vi "ETMF_ACP.vi"() -> ()   [LabVIEW 2019]
uses:
  <vilib>/Utility/error.llb/DialogType.ctl
  <vilib>/DAQmx/write.llb/DAQmx Write (Digital Bool 1Line 1Point).vi
  fd73fc79-9649-4217-8a97-07a7e50f329a.vi
  <vilib>/DAQmx/write.llb/DAQmx Write (Counter Frequency 1Chan 1Samp).vi
  df924464-8897-43aa-8929-2e0273e3eba3.vi
  1855413f-7d1b-4c6c-a6c5-1397daead511.vi
  7b2d4e1c-e7fc-4a66-bc21-bd6d40681ed8.vi
  <vilib>/numeric/Random Number (Range) DBL.vi
  <vilib>/DAQmx/miscellaneous.llb/DAQmx Fill In Error Info.vi
  varGlobal.vi
  <vilib>/DAQmx/create/channels.llb/DAQmx Create Channel (CO-Pulse Generation-Frequency).vi
  <vilib>/DAQmx/configure/timing.llb/DAQmx Timing (Implicit).vi
  <vilib>/addons/control/pid/pid.llb/PID (DBL).vi
  <vilib>/addons/control/pid/pid.llb/PID Gain Schedule (DBL).vi
  <vilib>/addons/control/pid/pid.llb/PID Advanced (DBL).vi
  <vilib>/Utility/file.llb/Write Delimited Spreadsheet (string).vi
  <instrlib>/Agilent 34970/Agilent 34970.lvlib
  <resource>/objmgr/daqmx.rc
  <vilib>/addons/control/pid/NI_PID_pid.lvlib
  <instrlib>/Yokogawa WT200 Series/Yokogawa WT200 Series.lvlib
  <instrlib>/Agilent 681x Series/Agilent 681x Series.lvlib
  48f1d8f6-73b3-4136-b681-12122d971459.vi
  <vilib>/ptbypt/NI_PtbyPt.lvlib
panel:
  out "SPs_Filtro":T1
  in  "Res_TempME":bool
  in  "INC_TempME":bool
  in  "ct_TempME":dbl
  in  "vecTempME":dbl[](array[numeric])
  out "ss_ceval":bool
  in  "vec_CEVAL":dbl[](array[numeric])
  in  "Res_CEVAL":bool
  in  "INC_CEVAL":bool
  in  "ct_CEVAL":dbl
  in  "increment":bool
  in  "ct_Estufa":dbl
  in  "vecEstufa":dbl[](array[numeric])
  in  "reset":bool
  out "PV_MI":dbl
  out "SP_Pwr":i32
  out "iter":i32
  out "Msg Erro":string
  out "error out Pt100":errorcluster
  out "error out TC":errorcluster
  in  "Tab Control":T2(tab)
  out "LIM SS":bool
  out "STEADY?":bool
  in  "TBR (min)":u32=10
  in  "Ts":dbl=1.0
  out "Time":dbl=300.0 format="%<%H:%M:%S>t"
  in  "Logfile_Estufa":string="medsForno"
  in  "Estufa_ON":bool=TRUE
  in  "Frequency":dbl=1.0 min=1.0 max=1.0 format="%.6f"
  in  "PID gains":T3={"proportional gain (Kc)"=39.6, "integral time (Ti, min)"=14.617, "derivative time (Td, min)"=0.0} {"derivative time (Td, min)" format="%.3f"; "integral time (Ti, min)" format="%.3f"; "proportional gain (Kc)" format="%.6f"}
  out "Process variable and Setpoint":cluster{"initial PV":dbl, "SP:":dbl}(graph)
  out "MV":dbl(graph)
  in  "SP:":dbl(slide)=60.0 min=0.0 max=0.0 scale=25.0..80.0
  out "PT100_CH9":dbl
  out "PT100_CH4":dbl
  out "Iteration":i32
  out "Duty Cycle":sgl=0.1 min=0.1 max=99.9 format="%#_6f"
  out "PV":dbl
  in  "STOP":bool
  out "Continue":bool
  in  "Manual":bool
  out "Pinv":u16
  out "DCBus":u16
  out "Vel Real":u16
  out "Chart_velo":cluster{"V(A)":dbl, "V(B)":dbl}(graph)
  in  "Tab Control 3":enum32{"Tensões", "Correntes", "Potências"}(tab)
  out "Chart_tensao":T4(graph)
  out "Chart_cur":T5(graph)
  out "Chart_power":T6(graph)
  out "pwr_cluster":T7
  out "cur_cluster":T8
  out "volt_cluster":T9
  in  "Tempo de integração (s)":u32=5 min=1 max=60 step=1
  in  "Realiza medição WT230":bool=TRUE
  in  "Medição contínua? WT230":bool=TRUE
  in  "Parâmetros serial":T10={"Serial VCC"="COM7", "timeout"=2, "baud rate"=600, "flow control"=0, "data bits"=8, "parity"=enum."None", "stop bits"=10, "termination char"=FALSE} {"stop bits" items=["1.0"=10, "1.5"=15, "2.0"=20]; "flow control" items=["None", "XON/XOFF", "RTS/CTS", "XON/XOFF & RTS/CTS", "DTR/DSR", "XON/XOFF & DTR/DSR"]}
  in  "Velocidade (RPM)":u16 min=1000 max=5000 step=100
  in  "Mensagem":T11(ring)=enum."Read power"
  in  "Limite de corrente":dbl min=0.0 max=0.31 step=0.01 format="%.4f"
  in  "Limite de tensão":dbl=24.0 min=0.0 max=36.0 step=0.5 format="%.4f"
  in  "Seta carga":bool
  in  "Enviar velocidade":bool
  in  "Envia mensagem":bool
  in  "Parar motor":bool
  out "Tradução":string
  out "Resposta":string
  in  "Liga Fonte":bool
  out "Corrente de saída":dbl format="%.4f"
  out "Tensão de saída":dbl format="%.4f"
  out "t":dbl
  in  "Logfile_Watt":string="medsWatt"
  in  "Logfile_Freio":string="medsFreio"
  in  "Tab Control 9":enum32{"COMP_EVAL", "POWER MAP"}(tab)
  out "SP_Vel":i32
  out "CP EV ok":bool
  in  "Skip":bool
  in  "bypass":bool
  in  "teste":bool
  in  "Ts MI":dbl=0.1
  out "MV_MI":dbl=5.583364480052211
  out "Condição Atual":string
  in  "Condicao para teste":T12(ring)
  in  "Logfile_ETMI":string="medsETMI"
  in  "Start EV?":bool
  out "Grafico_MI":cluster{"PV_MI":dbl, "MV_ME":sgl}(graph)
  in  "Ganhos PI do Gain Scheduling":T13(array[cluster])=[{"PID Parameters"={"Kc"=0.00026, "  Ti"=0.027, " Td"=0.0}, "Max PV"=490.0}, {"PID Parameters"={"Kc"=0.00027, "  Ti"=0.037, " Td"=0.0}, "Max PV"=690.0}, {"PID Parameters"={"Kc"=0.00019, "  Ti"=0.024, " Td"=0.0}, "Max PV"=900.0}] {"Max PV" format="%#.2f"; "PID Parameters"."Td" format="%#.3g"; "PID Parameters"."Ti" format="%#.3g"; "PID Parameters"."Kc" format="%#.5f"}
  out "Ganho atual do PI MI":T3={"proportional gain (Kc)"=100.0, "integral time (Ti, min)"=0.0, "derivative time (Td, min)"=0.0} {"derivative time (Td, min)" format="%.3f"; "integral time (Ti, min)" format="%.3f"; "proportional gain (Kc)" format="%.5f"}
  out "Graf_MV_MI":dbl(graph)
  out "MV_MIC":dbl format="%.2f"
  out "MV_C5":dbl format="%.2f"
  out "MV_L1":dbl format="%.2f"
  out "MV_C1":dbl format="%.2f"
  in  "Tab Control 10":enum32{"C1", "L1", "C5", "MIC"}(tab)
  in  "Gains_C1":T3={"proportional gain (Kc)"=232.52, "integral time (Ti, min)"=14.8, "derivative time (Td, min)"=0.0} {"derivative time (Td, min)" format="%.3f"; "integral time (Ti, min)" format="%.3f"; "proportional gain (Kc)" format="%.6f"}
  in  "Gains_L1":T3={"proportional gain (Kc)"=302.56, "integral time (Ti, min)"=7.42, "derivative time (Td, min)"=0.0} {"derivative time (Td, min)" format="%.3f"; "integral time (Ti, min)" format="%.3f"; "proportional gain (Kc)" format="%.6f"}
  in  "Gains_C5":T3={"proportional gain (Kc)"=249.72, "integral time (Ti, min)"=4.7, "derivative time (Td, min)"=0.0} {"derivative time (Td, min)" format="%.3f"; "integral time (Ti, min)" format="%.3f"; "proportional gain (Kc)" format="%.6f"}
  in  "Gains_MIC":T3={"proportional gain (Kc)"=259.498, "integral time (Ti, min)"=6.23, "derivative time (Td, min)"=0.0} {"derivative time (Td, min)" format="%.3f"; "integral time (Ti, min)" format="%.3f"; "proportional gain (Kc)" format="%.6f"}
  in  "TBRMF(min)":u32=10
  out "PV_MIC":dbl
  out "MV_ME":sgl=0.1 min=0.1 max=99.9 format="%#_6f"
  in  "Start PMAP?":bool
  in  "Logfile_ETME":string="medsETME"
  in  "Ts ME":dbl=1.0
  out "PW MP ok":bool
  out "STEADY MF?":bool
  out "Final Ensaio":bool
  out "LIM SS MF":bool
  in  "Tab Control 8":enum32{"C1", "L1", "C5", "MIC"}(tab)
  out "GME_C1":cluster{"SP_C1":dbl, "TP 1":dbl, "SP_F":dbl}(graph)
  out "Graf_MV_C1":dbl(graph)
  out "GME_L1":cluster{"SP_L1":dbl, "TP 10":dbl, "SP_F":dbl}(graph)
  out "Graf_MV_L1":dbl(graph)
  out "GME_C5":cluster{"SP_C5":dbl, "TP 12":dbl, "SP_F":dbl}(graph)
  out "Graf_MV_C5":dbl(graph)
  out "GME_MIC":cluster{"SP_MIC":dbl, "TP 13":dbl, "SP_F":dbl}(graph)
  out "Graf_MV_MIC":dbl(graph)
  in  "Tab Control 11":enum32{"C1", "L1", "C5", "MIC"}(tab)
  in  "zF_C1":dbl=0.75 min=0.0 max=1.0 step=0.1
  out "zF_C1_i":dbl(knob)=0.75 min=0.0 max=0.99 step=0.1 scale=0.0..1.0
  in  "SP_C1":dbl=70.0 caption="SP C011:" min=0.0 max=0.0
  in  "zF_L1":dbl=0.75 min=0.0 max=1.0 step=0.1
  out "zF_L1_i":dbl(knob)=0.75 min=0.0 max=0.99 step=0.1 scale=0.0..1.0
  in  "SP_L1":dbl=70.0 caption="SP L100:" min=0.0 max=0.0
  in  "zF_C5":dbl=0.75 min=0.0 max=1.0 step=0.1
  out "zF_C5_i":dbl(knob)=0.75 min=0.0 max=0.99 step=0.1 scale=0.0..1.0
  in  "SP_C5":dbl=70.0 caption="SP C504:" min=0.0 max=0.0
  in  "zF_MIC":dbl=0.75 min=0.0 max=1.0 step=0.1
  out "zF_MIC_i":dbl(knob)=0.75 min=0.0 max=0.99 step=0.1 scale=0.0..1.0
  in  "SP_MIC":dbl=70.0 caption="SP MIC:" min=0.0 max=0.0
  in  "Tab Control 2":enum32{"1-7", "8-15"}(tab)
  out "G. TP 1":cluster{dbl, "index":i32}(graph)
  out "TP 1":dbl
  out "TP 2":dbl
  out "G. TP 2":cluster{dbl, "index":i32}(graph)
  out "G. TP 3":cluster{dbl, "index":i32}(graph)
  out "TP 3":dbl
  out "G. TP 5":cluster{dbl, "index":i32}(graph)
  out "TP 5":dbl
  out "G. TP 6":cluster{dbl, "index":i32}(graph)
  out "TP 6":dbl
  out "G. TP 7":cluster{dbl, "index":i32}(graph)
  out "TP 7":dbl
  out "G. TP 8":cluster{dbl, "index":i32}(graph)
  out "TP 8":dbl
  out "G. TP 10":cluster{dbl, "index":i32}(graph)
  out "TP 10":dbl
  out "G. TP 11":cluster{dbl, "index":i32}(graph)
  out "TP 11":dbl
  out "G. TP 12":cluster{dbl, "index":i32}(graph)
  out "TP 12":dbl
  out "G. TP 13":cluster{dbl, "index":i32}(graph)
  out "TP 13":dbl
  out "G. TP 15":cluster{dbl, "index":i32}(graph)
  out "TP 15":dbl
  in  "Logfile_TPs":string="medsETMA"
  in  "Logfile_Dina":string="medsYDin"
  out "Chart Temperatura":cluster{dbl, dbl, dbl, dbl, dbl, dbl}(graph)={21.505, 22.941, 24.092, 23.94, 23.972, 20.648}
  out "temp pts":T14
  in  "Tab Control 5":enum32{"CONFIG", "COM"}(tab)
  in  "Configurações":T15={"Tipo de tensão"=enum."AC", "Tensão (V)"=0.0, "Limite de corrente (A)"=0.0, "Frequência (Hz)"=60.0, "Limite de Potência (kW)"=0.0} {"Limite de Potência (kW)" min=0.0 max=300.0; "Frequência (Hz)" min=43.0 max=63.0; "Limite de corrente (A)" min=0.0 max=15.5; "Tensão (V)" min=0.0 max=300.0}
  in  "VISA name (EEC)":refnum<visa-resource-name>="Extech"
  in  "Timeout":i32=10000
  in  "RST*":bool
  in  "error in (EEC)":errorcluster
  out "error Out (EEC)":errorcluster
  in  "Logfile_EEC":string="medsZeec"
  in  "Tab Control 7":enum32{"VOLT", "CURR", "PWR"}(tab)
  out "EEC_VOLT":cluster{"Peak Current":dbl}(graph)
  out "EEC_CURR":cluster{"Peak Current":dbl}(graph)
  out "EEC_PWR":cluster{"Peak Current":dbl}(graph)
  in  "Tab Control 6":enum32{"VOLT", "CURR", "PWR"}(tab)
  out "ACP_VOLT":cluster{"Peak Current":dbl}(graph)
  out "ACP_CUR":T16(graph)
  out "ACP_PWR":T17(graph)
  out "PwrMeas":cluster{"Total Power":dbl, "Power Factor":dbl}
  out "VolMeas":cluster{"AC + DC RMS Voltage":dbl}
  out "CurMeas":T18
  in  "Tab Control 4":enum32{"CONFIG", "PROT", "COM"}(tab)
  in  "Muda tensao":bool
  in  "Triggered Voltage Amplitude (V)":dbl=1.0 min=0.0 max=300.0 format="%#.4g"
  in  "Trigger Delay (s)":dbl=10.0 format="%#.5g"
  in  "Period (s)":dbl=10.0 format="%#.4g"
  in  "Pulse Characteristic":u16(ring) items=["Duty Cycle", "Pulse Width"]
  in  "Pulse Count":dbl=1.0 format="%#.4g"
  in  "Pulse Characteristic Value (%)":dbl=100.0 min=0.0 max=100.0 format="%#.4g"
  in  "Voltage Mode (0: Fix)":u16(ring) items=["Fixed", "Step", "Pulse", "List"]
  in  "Voltage Amplitude (1.0 V)":dbl min=0.0 max=300.0 format="%#.4g"
  in  "RMS Current Limit (1 A)":dbl=0.3 min=0.1 max=10.0 format="%#.4g"
  in  "Peak Current Limit (13 A)":dbl=0.5 min=0.1 max=20.0 format="%#.4g"
  in  "Output Waveform Type (0: Sinusoid)":u16(ring) items=["Sinusoid", "Square", "Clipped Sinusoid", "User Specified"]
  in  "Output Frequency (60 Hz)":dbl=60.0 format="%#.4g"
  in  "Serial Configuration":T19={"Baud Rate"=9600, "Parity"=0, "Data Bits"=8} {"Data Bits" items=["7"=7, "8"=8]; "Parity" items=["None", "Odd", "Even", "Mark", "Space"]; "Baud Rate" items=["300"=300, "600"=600, "1200"=1200, "2400"=2400, "4800"=4800, "9600"=9600]}
  out "error out (6812B)":errorcluster
  in  "VISA  name (6812B)":refnum<visa-resource-name>="6812B"
  in  "Logfile_6812B":string="meds6812B"
  out "EEC_OUT":T20
  # "Controle de Temperatura da Estufa"
  # "Geral"
  # "Respostas do Sistema em Malha Fechada"
  # "Controles"
  # "Medidas"
  # "Freio"
  # "Wattímetro WT230 Yokogawa"
  # "Controles:"
  # "Log File:"
  # "Controles"
  # "Medidas"
  # "Respostas temporais"
  # "Medidas"
  # "Inversor de Frequência"
  # "Controles"
  # "Comandos"
  # "Velocidade atual medida pelo inversor (RPM)"
  # "Tensão de barramento medida pelo inversor (V)"
  # "Parâmetros Serial"
  # "Controle Automático do Ensaio do Térmico"
  # "Log File:"
  # "Condição de Operação"
  # "Medidas do Sistema"
  # "Parâmetros de Controle"
  # "Log File:"
  # "Limites térmicos:"
  # "Amostragem:"
  # "Assentamento:"
  # "Parâmetros de Controle"
  # "Medidas"
  # "Filtro"
  # "+Agressivo"
  # "+Agressivo"
  # "+Agressivo"
  # "+Agressivo"
  # "Temperaturas dos Termopares"
  # "Log file:"
  # "Legenda:"
  # "TP 1: Termopar do Capacitor C011"
  # "TP 3: Termopar do Choke L001"
  # "TP 2: Termopar do Capacitor C009"
  # "TP 5: Termopar do Capacitor C006"
  # "TP 6: Termopar do Fusível F002"
  # "TP 7: Termopar do Conector CN204"
  # "TP 8: Termopar do CI SMPS IC 100"
  # "TP 10: Termopar do Indutor L100"
  # "TP 11: Termopar do Capacitor C112"
  # "TP 12: Termopar do Capacitor C504"
  # "TP 13: Termopar do Microcontrolador IC601"
  # "TP 15: Termopar do Dissipador"
  # "Temperaturas do Motor/Freio"
  # "Log file:"
  # "Fontes de Corrente Alternada Programáveis"
  # "Keysight 6812B"
  # "Medidas:"
  # "Extech EEC-6510"
  # "Medidas:"
  # "Trigger:"
  # "Forma de Onda"
  # "Proteção contra Sobrecorrente"
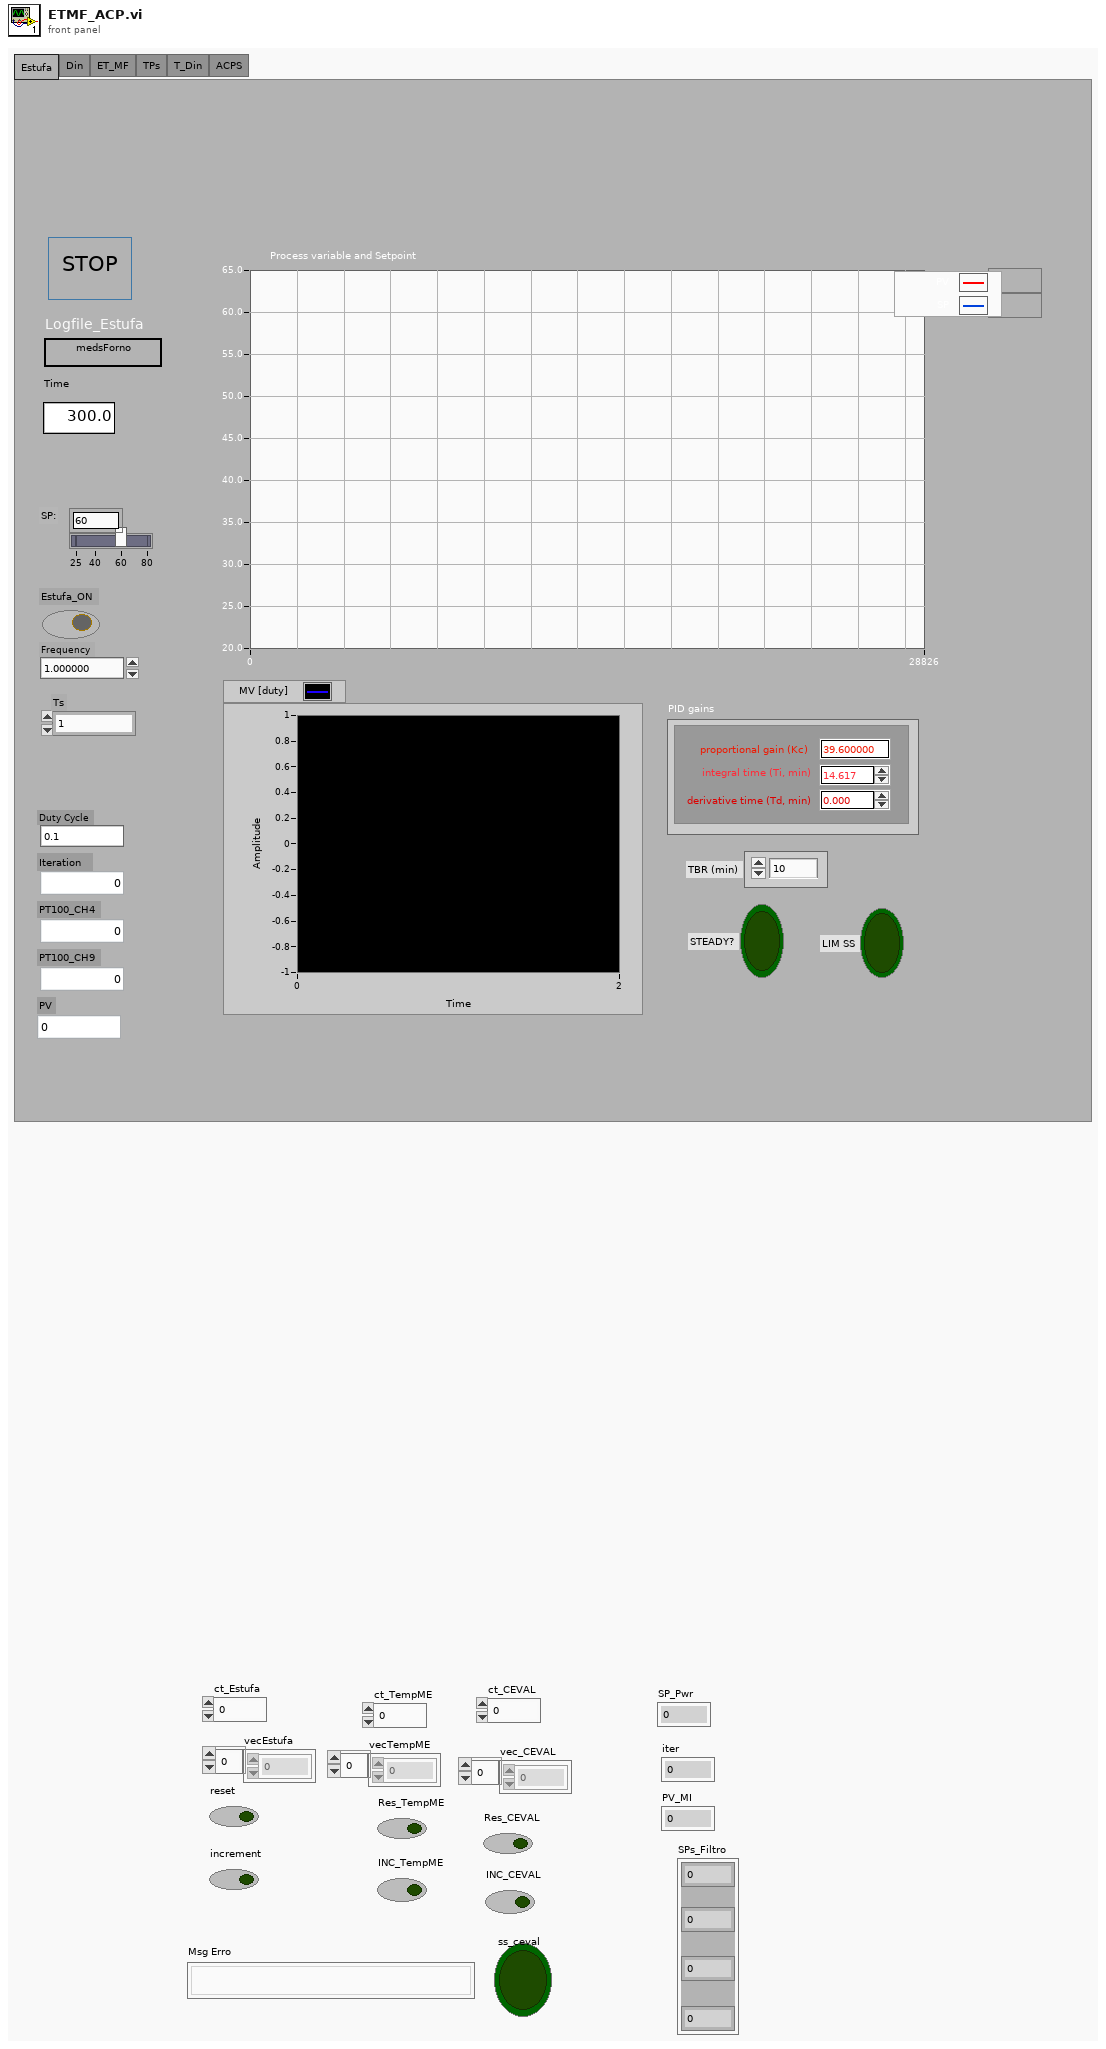
[diagram p1: front panel]
types:
  T1 = cluster{"SP_F":dbl, "SP_F":dbl, "SP_F":dbl, "SP_F":dbl}
  T2 = enum32{"Estufa", "Din", "ET_MF", "TPs", "T_Din", "ACPS"}
  T3 = cluster{"proportional gain (Kc)":dbl, "integral time (Ti, min)":dbl, "derivative time (Td, min)":dbl}
  T4 = cluster{"V(A)":dbl, "V(B)":dbl, "V(E)":dbl, "V(E) 2":dbl}
  T5 = cluster{"I(A)":dbl, "I(B)":dbl, "I(E)":dbl, "I(E) 2":dbl}
  T6 = cluster{"PC(A)":dbl, "PC(B)":dbl, "PC(T)":dbl, "PL(A)":dbl, "PL(B)":dbl, "PL(T)":dbl, "PC(E)":dbl, "PL(E)":dbl, "PL(E) 2":dbl}
  T7 = cluster{"PC(A)":dbl, "PC(B)":dbl, "PC(T)":dbl, "PL(A)":dbl, "PL(B)":dbl, "PL(T)":dbl, "PC(E)":dbl, "PL(E) - 6812B":dbl, "PL(E) - Extech":dbl}
  T8 = cluster{"I(A)":dbl, "I(B)":dbl, "I(E) - 6812B":dbl, "I(E) - Extech":dbl}
  T9 = cluster{"V(A)":dbl, "V(B)":dbl, "V(E) - 6812B":dbl, "V(E) - Extech":dbl}
  T10 = cluster{"Serial VCC":refnum<visa-resource-name>, "timeout":u32, "baud rate":u32, "flow control":u16, "data bits":u16, "parity":enum16{"None", "Odd", "Even", "Mark", "Space"}, "stop bits":u16, "termination char":bool}
  T11 = enum16{"Read set speed", "Read operation status", "Read power", "Read starting trials", "Read bus voltage", "Read temperature", "Read power limitation", "Read PWM mode", "Read PWM frequency", "Read real speed"}
  T12 = enum16{"3500RPM@675W", "3500RPM@720W", "3500RPM@775W", "3500RPM@830W", "3500RPM@885W"}
  T13 = cluster{"PID Parameters":cluster{"Kc":dbl, "  Ti":dbl, " Td":dbl}, "Max PV":dbl}[]
  T14 = cluster{"t1 freio":dbl, "t2 bob 1":dbl, "t5 bob 2":dbl, "t4 estat 2":dbl, "t3 estat 1":dbl, "t6 amb":dbl}
  T15 = cluster{"Tipo de tensão":enum16{"AC", "DC", "AC/DC"}, "Tensão (V)":dbl, "Limite de corrente (A)":dbl, "Frequência (Hz)":dbl, "Limite de Potência (kW)":dbl}
  T16 = cluster{"Peak Current":dbl, "AC RMS Current":dbl}
  T17 = cluster{"Reactive Power":dbl, "Apparent Power":dbl}
  T18 = cluster{"Peak Current":dbl, "AC + DC RMS Cur":dbl}
  T19 = cluster{"Baud Rate":u32, "Parity":u16, "Data Bits":u16}
  T20 = cluster{"Frequency":dbl, "AC Voltage":dbl, "Current":dbl, "Power":dbl, "Power Factor":dbl}
  T21 = enum16{"Start Comm.", "End Comm.", "Wait", "Send Static Message", "Set Speed"}
  T22 = enum8{"Enabled", "Disabled", "Disabled and Grayed Out"}
  T23 = enum16{"Thermocouple", "Thermistor", "RTD", "4-Wire RTD", "Default (Last)"}
  T24 = cluster{"Peak Current":dbl, "AC + DC RMS Current":dbl}
  T25 = cluster{"Frequency":dbl, "AC Voltage":dbl, "Current":dbl, "Power":dbl, "Power Factor":dbl, "Timer":dbl, "a":dbl, "b":dbl, "c ":dbl, "d":dbl, "e":dbl, "f":dbl, "g":dbl}
  T26 = cluster{"Frequency":dbl, "AC Voltage":dbl, "Current":dbl, dbl, "Power Factor":dbl}
  T27 = cluster{"V(A)":dbl, "I(A)":dbl, "V(B)":dbl, "I(B)":dbl, "PC(A)":dbl, "PC(B)":dbl, "PC(T)":dbl, "PL(T)":dbl, "PL(B)":dbl, "PL(A)":dbl, "V(E)":dbl, "PL(E)":dbl, "PC(E)":dbl, "I(E)":dbl, "t":dbl}
  T28 = cluster{"V(A)":dbl, "V(B)":dbl, "V(E)":dbl, "AC Voltage":dbl}
  T29 = cluster{"I(A)":dbl, "I(B)":dbl, "I(E)":dbl, "Current":dbl}
  T30 = cluster{"output":dbl, "output":dbl, "output":dbl, "PL(A)":dbl, "PL(B)":dbl, "PL(T)":dbl, "output":dbl, "PL(E)":dbl, "Power":dbl}
  T31 = typedef "DialogType.ctl" = u16
  T32 = cluster{"TP 1":dbl, "TP 10":dbl, "TP 12":dbl, "TP 13":dbl}
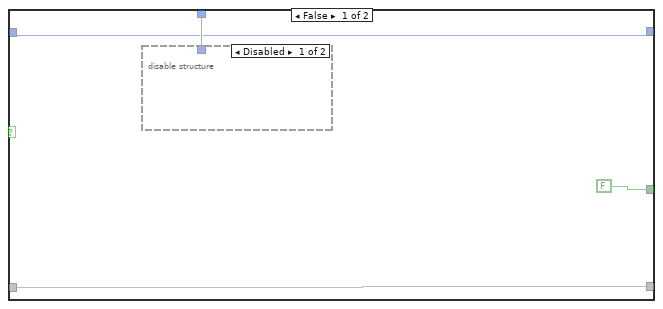
[diagram p2: hidden frame]
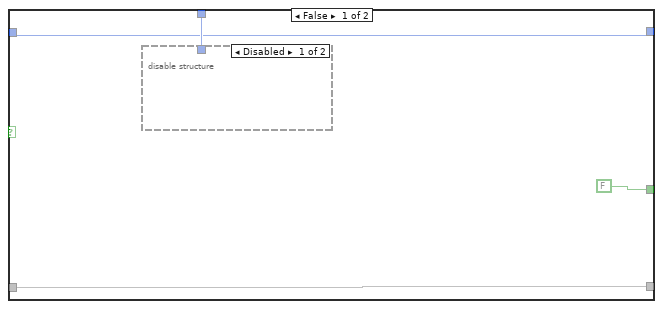
[diagram p4: hidden frame]
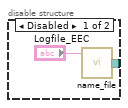
[diagram p9: hidden frame]
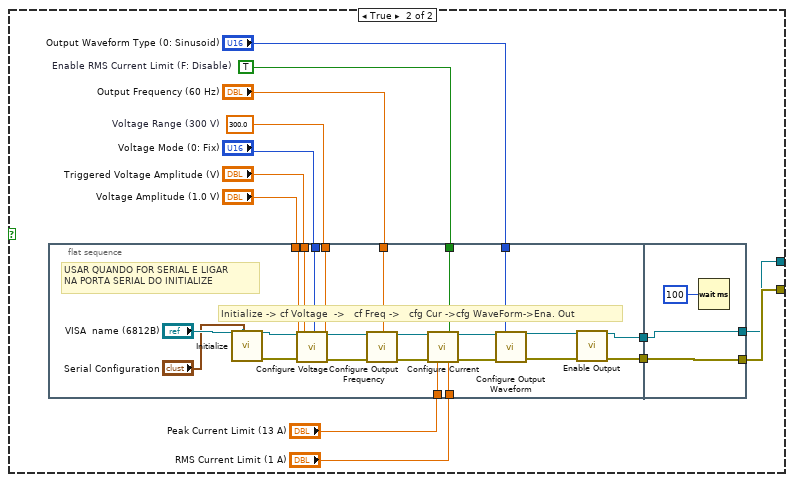
[diagram p11: hidden frame]
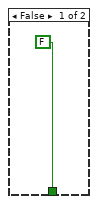
[diagram p12: hidden frame]
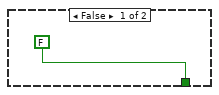
[diagram p13: hidden frame]
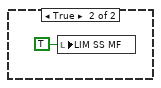
[diagram p17: hidden frame]
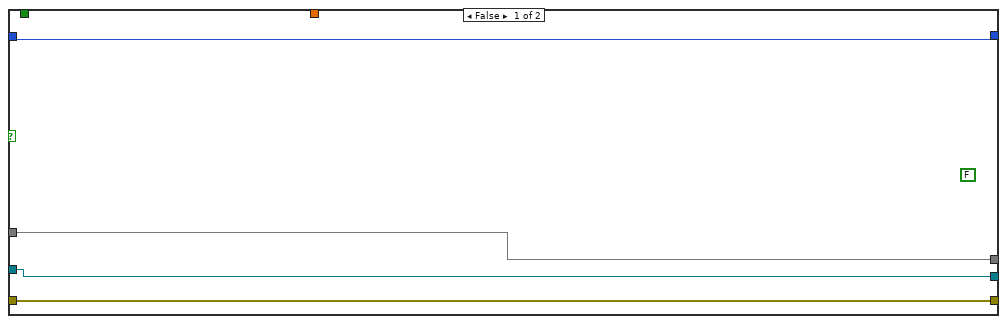
[diagram p18: hidden frame]
diagram:
  # "Se os últimos três valores medidos consecutivamente num intervalo de TBR [minutos] \nestiverem dentro do limite desejado, então a condição é true."
  n1 = flat-sequence {
    tunnel: [w81] -> w14
    tunnel: [w80] -> w13
    tunnel: [w77] -> w12
    tunnel: [w75] -> w11
    tunnel: [w73] -> w10
    tunnel: [w71] -> w9
    tunnel: [w69] -> w8
    tunnel: [w64] -> w7
    tunnel: [w51] -> w6
    tunnel: [w50] -> w5
    tunnel: [w56] -> w4
    tunnel: [w38] -> w3
    tunnel: [w29] -> w2
    tunnel: [w28] -> w1
    tunnel: w14 -> [w302]
    tunnel: w13 -> [w321]
    tunnel: w12 -> [w320]
    tunnel: w11 -> [w315]
    tunnel: w10 -> [w306]
    tunnel: w9 -> [w298]
    tunnel: w8 -> [w296]
    tunnel: w7 -> [w293]
    tunnel: w6 -> [w290]
    tunnel: w5 -> [w289]
    tunnel: w4 -> [w288]
    tunnel: w3 -> [w286]
    tunnel: w2 -> [w271]
    tunnel: w1 -> [w270]
    frame #0 {
      w20 = 0.0 ("Graf_MV_C1")
      w21 = cluster{"SP_C1":dbl, "TP 1":dbl, "SP_F":dbl} {"SP_C1"=0.0, "TP 1"=0.0, "SP_F"=0.0} ("GME_C1")
      w24 = 0.0 ("counter")
      w39 = FALSE ("STOP_GERAL")
      w23 = FALSE ("Auto Enab?")
      w65 = 0.0 ("Temperature 1")
      w22 = 0.0 ("PC(E)")
      w41 = u16 0 ("Velocidade (RPM)")
      w70 = TRUE ("Realiza medição WT230")
      # "Define o tamanho do gauge e do controle do zero do filtro 2 DOF"
      # "Inicia vetor do algoritmo de leituras da estufa e do ceval"
      # "Zera contador do contador de leituras de temp da estufa"
      # "Seta velocidade do motor para o ensaio"
      # "Inicializando as variáveis chart do Wattímetro WT230:"
      # "Inicializando parâmetros controle fonte Lambda:"
      # "Inicializa a fonte Keysight 6812B que liga o ventilador"
      # "Liga fonte Lambda e seta carga para zero"
      # "Estabelece Comunicação com o Inversor"
      # "Inicializando as medidas elétricas da fonte EEC 6510"
      # "Inicializando as medidas elétricas Wattímetro WT330"
      # "Inicializando as variáveis do Agilent 34972A:"
      # "Inicializando as variaveis das malhas de controle da estufa, da carga e das medidores de regime permanente"
      # "Inicializando as medidas elétricas da fonte 6812B"
      # "Inicia Wattímetro e liga relé SSR:"
      # "Controle Automático, Inversor e Fonte  Lambda desligados:"
      # "Zera variaveis lidas pelo inversor e a iteracao"
      # "Declaração variáveis de controle e de erro"
      n2 = case shown="True" TRUE {
        tunnel: [FALSE w228] -> w58
        frame False {
        }
        frame True {
          n3 = flat-sequence {
            tunnel: [w233] -> w229
            tunnel: [w236] -> w230
            tunnel: w229 -> [w236]
            tunnel: [w238] -> w231
            tunnel: w230 -> [w238]
            tunnel: [w241] -> w232
            tunnel: w231 -> [w241]
            tunnel: w232 -> [w246]
            tunnel: [TRUE ("STOP")] -> w228
            frame #0 {
              w234 = refnum<k21> "alimentacao_inversor"  # DAQmx Task Name
              n4 = call <vilib>:"DAQmx Start Task.vi"("task/channels in"=w234) -> ("task out"=w233:refnum<k21>)  [unwired: 13 in, 1 out]
              n5 = call-poly <vilib>:"DAQmx Write.vi"("task/channels in"=w233, "data"=TRUE) -> ()  [unwired: 11 in, 3 out]
            }
            frame #1 {
              # "era 3000"
              n6 = Wait (ms)(milliseconds to wait=u32 100) -> ()  [unwired: 1 out]
            }
            frame #2 {
              # "inicia comunicacao"
              n7 = call "Serial_control.vi"("Função"=T21."Start Comm.", "comm cluster"="Parâmetros serial") -> ()  [unwired: 3 in, 4 out]
            }
            frame #3 {
              # "seta velocidade igual a zero"
              n8 = local read "Parâmetros serial"() -> (w243:T10)
              n9 = call "Serial_control.vi"("Enviar número"=u16 0, "Função"=T21."Set Speed", "comm cluster"=w243) -> ()  [unwired: 2 in, 4 out]
            }
            frame #4 {
              n10 = call <vilib>:"DAQmx Clear Task.vi"("task in"=w246) -> ()  [unwired: 14 in, 1 out]
            }
          }
        }
      }
      n11 = flat-sequence {
        tunnel: [w85] -> w18
        tunnel: [w85] -> w17
        tunnel: [w85] -> w16
        tunnel: [w85] -> w15
        tunnel: w18 -> [w103]
        tunnel: w17 -> [w102]
        tunnel: w16 -> [w100]
        tunnel: w15 -> [w101]
        frame #0 {
          w85 = 1.0
          n12 = disable-structure shown="Disabled" {
            disable-tunnel: [w94 _] -> _
            disable-tunnel: [w91 _] -> _
            disable-tunnel: [w89 _] -> _
            disable-tunnel: [w86 _] -> _
            frame Disabled {
              w88 = 60.0 ("x")
              # "Ti_C1 em seg"
              n13 = local read "Gains_MIC"() -> (w98:T3)
              n14 = local read "Gains_C5"() -> (w97:T3)
              n15 = local read "Gains_C1"() -> (w95:T3)
              n16 = local read "Gains_L1"() -> (w96:T3)
              n17 = Unbundle By Name(w98) -> ("integral time (Ti, min)"=w87:dbl)  [unwired: 1 out]
              n18 = Unbundle By Name(w97) -> ("integral time (Ti, min)"=w90:dbl)  [unwired: 1 out]
              n19 = Unbundle By Name(w95) -> ("integral time (Ti, min)"=w93:dbl)  [unwired: 1 out]
              n20 = Unbundle By Name(w96) -> ("integral time (Ti, min)"=w92:dbl)  [unwired: 1 out]
              n21 = Multiply(x=w88, y=w93) -> (x*y=w94:dbl)
              n22 = Multiply(x=w88, y=w92) -> (x*y=w91:dbl)
              n23 = Multiply(x=w88, y=w90) -> (x*y=w89:dbl)
              n24 = Multiply(x=w88, y=w87) -> (x*y=w86:dbl)
            }
            frame Enabled {
            }
          }
        }
        frame #1 {
          w99 = 0.85 ("zF_C1")
          # "Inicialmente, tau_d = Ti/8"
          # "Control"
          # "Gauge"
          n25 = property on="zF_C1_i" class="Knob (strict)"("Scale.Maximum"=w103) -> ()  [unwired: 2 in, 2 out]
          n26 = property on="zF_L1_i" class="Knob (strict)"("Scale.Maximum"=w102) -> ()  [unwired: 2 in, 2 out]
          n27 = property on="zF_C5_i" class="Knob (strict)"("Scale.Maximum"=w100) -> ()  [unwired: 2 in, 2 out]
          n28 = property on="zF_MIC_i" class="Knob (strict)"("Scale.Maximum"=w101) -> ()  [unwired: 2 in, 2 out]
          n29 = property on="zF_C1" class="DigNum (strict)"("Maximum"=w103) -> ()  [unwired: 2 in, 2 out]
          n30 = property on="zF_L1" class="DigNum (strict)"("Maximum"=w102) -> ()  [unwired: 2 in, 2 out]
          n31 = property on="zF_C5" class="DigNum (strict)"("Maximum"=w100) -> ()  [unwired: 2 in, 2 out]
          n32 = property on="zF_MIC" class="DigNum (strict)"("Maximum"=w101) -> ()  [unwired: 2 in, 2 out]
          n33 = property on="zF_C1" class="DigNum (strict)"("Value"=w99) -> ()  [unwired: 2 in, 2 out]
          n34 = property on="zF_L1" class="DigNum (strict)"("Value"=w99) -> ()  [unwired: 2 in, 2 out]
          n35 = property on="zF_C5" class="DigNum (strict)"("Value"=w99) -> ()  [unwired: 2 in, 2 out]
          n36 = property on="zF_MIC" class="DigNum (strict)"("Value"=w99) -> ()  [unwired: 2 in, 2 out]
        }
      }
      n37 = disable-structure shown="Disabled" {
        disable-tunnel: [w107 _] -> w51
        disable-tunnel: [w106 _] -> w50
        frame Disabled {
          # "Inicializa  e configura a saída da fonte EXTECH 6510 (que alimenta o inversor)"
          n38 = flat-sequence {
            tunnel: [w134] -> w123
            tunnel: [w133] -> w122
            tunnel: [w132] -> w121
            tunnel: [w131] -> w120
            tunnel: [w125] -> w119
            tunnel: w123 -> [w142]
            tunnel: w122 -> [w139]
            tunnel: w121 -> [w141]
            tunnel: w120 -> [w140]
            tunnel: w119 -> [w138]
            tunnel: [w142] -> w118
            tunnel: [w141] -> w117
            tunnel: [w140] -> w116
            tunnel: [w137] -> w115
            tunnel: [w136] -> w114
            tunnel: w118 -> [w147]
            tunnel: w117 -> [w145]
            tunnel: w116 -> [w152]
            tunnel: w115 -> [w153]
            tunnel: w114 -> [w151]
            tunnel: [w144] -> w113
            tunnel: [w143] -> w112
            tunnel: w113 -> [w156]
            tunnel: w112 -> [w155]
            tunnel: [w156] -> w111
            tunnel: [w155] -> w110
            tunnel: w111 -> [w160]
            tunnel: w110 -> [w159]
            tunnel: [w158] -> w109
            tunnel: [w157] -> w108
            tunnel: [w161] -> w106
            tunnel: [w162] -> w107
            tunnel: w109 -> [w162]
            tunnel: w108 -> [w161]
            frame #0 {
              # "Inicializa"
              n39 = Unbundle By Name("Configurações") -> ("Tensão (V)"=w131:dbl, "Limite de corrente (A)"=w132:dbl, "Frequência (Hz)"=w134:dbl)  [unwired: 1 out]
              n40 = call "Inicializa_Reset (SubVI).vi"("error in (no error)"="error in (EEC)", "Reset"="RST*", "Timeout\n(10000 ms)"="Timeout", "VISA Refnum in"="VISA name (EEC)") -> ("error out"=w133:errorcluster, "Mensagem de erro"=→"Msg Erro":string, "VISA Refnum out"=w125:refnum<visa-resource-name>)  [unwired: 4 in, 1 out]
            }
            frame #1 {
              # "Aplica Range de tensão"
              # "Define Range"
              n41 = call "Define_Range (SubVI).vi"("Tensão (V)"=w140) -> ("Range X"=w135:i16)  [unwired: 10 in]
              n42 = call "Range_tensao(SubVI).vi"("error in (no error)"=w139, "Range"=w135, "VISA Refnum in"=w138) -> ("error out"=w137:errorcluster, "VISA Refnum out"=w136:refnum<visa-resource-name>)  [unwired: 7 in]
            }
            frame #2 {
              # "Envia tensão, freq e lim corrente"
              n43 = call "Tensao_AC (SubVI).vi"("error in (no error)"=w153, "Tensão (V)"=w152, "VISA Refnum in"=w151) -> ("error out"=w148:errorcluster, "VISA Refnum out"=w146:refnum<visa-resource-name>)  [unwired: 7 in]
              n44 = call "Frequência (SubVI).vi"("error in (no error)"=w148, "Frequência (Hz)"=w147, "VISA Refnum in"=w146) -> ("error out"=w150:errorcluster, "VISA Refnum out"=w149:refnum<visa-resource-name>)  [unwired: 7 in]
              n45 = call "Limite de corrente High (SubVI).vi"("error in (no error)"=w150, "Limite de corrente"=w145, "VISA Refnum in"=w149) -> ("error out"=w144:errorcluster, "VISA Refnum out"=w143:refnum<visa-resource-name>)  [unwired: 7 in]
            }
            frame #3 {
              n46 = Wait (ms)(milliseconds to wait=u32 500) -> ()  [unwired: 1 out]
            }
            frame #4 {
              # "Liga a saída"
              n47 = call "Power On.vi"("error in (no error)"=w160, "VISA Refnum in"=w159) -> ("error out"=w157:errorcluster, "VISA Refnum out"=w158:refnum<visa-resource-name>)  [unwired: 8 in]
            }
            frame #5 {
            }
          }
        }
        frame Enabled {
        }
      }
      n48 = case shown="True" w58 {
        tunnel: [FALSE ("STOP") w210] -> w52
        frame False {
        }
        frame True {
          n49 = flat-sequence {
            tunnel: [w212] -> w207
            tunnel: [w211] -> w204
            tunnel: [w216] -> w208
            tunnel: w207 -> [w216]
            tunnel: [w215] -> w205
            tunnel: w204 -> [w215]
            tunnel: [w219] -> w209
            tunnel: w208 -> [w219]
            tunnel: [w218] -> w206
            tunnel: w205 -> [w218]
            tunnel: w209 -> [w223]
            tunnel: w206 -> [w222]
            tunnel: [TRUE ("STOP")] -> w210
            frame #0 {
              # "Liga fonte"
              n50 = call <instrlib>:"GENie Config Output On-Off.vi"("Output ON"=TRUE, "VISA"=refnum<visa-resource-name> "Lambda" ("VISA name")) -> ("error out"=w211:errorcluster, "VISA out"=w212:refnum<visa-resource-name>)  [unwired: 8 in]
            }
            frame #1 {
              n51 = Wait (ms)(milliseconds to wait=u32 100) -> ()  [unwired: 1 out]
            }
            frame #2 {
              n52 = local write "Seta carga"(TRUE ("Seta carga")) -> ()
            }
            frame #3 {
              # "corrente igual a zero"
              n53 = call <instrlib>:"GENie Config Current Limit.vi"("error"=w222, "Current Limit"=0.0, "VISA"=w223) -> ()  [unwired: 7 in, 2 out]
            }
            frame #4 {
              n54 = local write "Seta carga"(FALSE ("Seta carga")) -> ()
              n55 = Wait (ms)(milliseconds to wait=u32 100) -> ()  [unwired: 1 out]
            }
            frame #5 {
            }
          }
        }
      }
      n56 = case shown="False" w52 {
        tunnel: [errorcluster {"status"=FALSE, "code"=0, "source"=""} ("error out") w166] -> w29
        tunnel: [w164 w165] -> w28
        frame False {
          n57 = local read "VISA  name (6812B)"() -> (w164:refnum<visa-resource-name>)
        }
        frame True {
          w171 = TRUE  # Enable RMS Current Limit (F: Disable)
          w170 = 300.0  # Voltage Range (300 V)
          n58 = flat-sequence {
            tunnel: "Output Frequency (60 Hz)" -> [w197]
            tunnel: "Voltage Mode (0: Fix)" -> [w195]
            tunnel: "RMS Current Limit (1 A)" -> [w193]
            tunnel: "Output Waveform Type (0: Sinusoid)" -> [w192]
            tunnel: "Voltage Amplitude (1.0 V)" -> [w191]
            tunnel: "Triggered Voltage Amplitude (V)" -> [w190]
            tunnel: w171 -> [w185]
            tunnel: w170 -> [w184]
            tunnel: "Peak Current Limit (13 A)" -> [w181]
            tunnel: [w179] -> w168
            tunnel: [w178] -> w167
            tunnel: w168 -> [w201]
            tunnel: w167 -> [w200]
            tunnel: [w201] -> w165
            tunnel: [w200] -> w166
            frame #0 {
              # "USAR QUANDO FOR SERIAL E LIGAR \nNA PORTA SERIAL DO INITIALIZE"
              # "Initialize -> cf Voltage  ->   cf Freq ->   cfg Cur ->cfg WaveForm->Ena. Out"
              n59 = call <instrlib>:"Initialize.vi"("Serial Configuration"="Serial Configuration", "VISA resource name"="VISA  name (6812B)") -> ("error out"=w196:errorcluster)  [unwired: 8 in, 1 out]
              n60 = call <instrlib>:"Configure Voltage.vi"("VISA resource name"="VISA  name (6812B)", "Triggered Voltage Amplitude (1.0 V)"=w190, "Voltage Range (300 V)"=w184, "Voltage Amplitude (1.0 V)"=w191, "Voltage Mode (0: Fix)"=w195, "error in (no error)"=w196) -> ("VISA resource name out"=w189:refnum<visa-resource-name>, "error out"=w188:errorcluster)  [unwired: 8 in]
              n61 = call <instrlib>:"Configure Output Frequency.vi"("VISA resource name"=w189, "Output Frequency (60 Hz)"=w197, "error in (no error)"=w188) -> ("VISA resource name out"=w198:refnum<visa-resource-name>, "error out"=w199:errorcluster)  [unwired: 11 in]
              n62 = call <instrlib>:"Configure Current.vi"("VISA resource name"=w198, "Enable RMS Current Limit (F: Disable)"=w185, "RMS Current Limit (1 A)"=w193, "error in (no error)"=w199, "Peak Current Limit (13 A)"=w181) -> ("VISA resource name out"=w187:refnum<visa-resource-name>, "error out"=w186:errorcluster)  [unwired: 9 in]
              n63 = call <instrlib>:"Configure Output Waveform.vi"("VISA resource name"=w187, "Output Waveform Type (0: Sinusoid)"=w192, "error in (no error)"=w186) -> ("VISA resource name out"=w183:refnum<visa-resource-name>, "error out"=w182:errorcluster)  [unwired: 11 in]
              n64 = call <instrlib>:"Enable Output.vi"("VISA resource name"=w183, "error in (no error)"=w182) -> ("VISA resource name out"=w179:refnum<visa-resource-name>, "error out"=w178:errorcluster)  [unwired: 12 in]
            }
            frame #1 {
              n65 = Wait (ms)(milliseconds to wait=u32 100) -> ()  [unwired: 1 out]
            }
          }
        }
      }
      n66 = local write "Realiza medição WT230"(w70) -> ()
      n67 = local write "Estufa_ON"(w70) -> ()
      n68 = local write "DCBus"(w41) -> ()
      n69 = local write "Iteration"(w41) -> ()
      n70 = local write "Pinv"(w41) -> ()
      n71 = local write "Velocidade (RPM)"(u16 0 ("Velocidade (RPM)")) -> ()
      n72 = local write "Limite de corrente"(0.0 ("Limite de corrente")) -> ()
      n73 = global write "varGlobal.vi" "STOP_GERAL"(w39) -> ()
      n74 = local write "Enviar velocidade"(w39) -> ()
      n75 = local write "Seta carga"(w39) -> ()
      n76 = local write "Liga Fonte"(w39) -> ()
      n77 = local write "Manual"(w39) -> ()
      n78 = local write "Limite de tensão"(24.0 ("Limite de tensão")) -> ()
      n79 = local write "ct_Estufa"(w24) -> ()
      n80 = Initialize Array(-999.0 ("element"), 3 ("dimension size")) -> (w34:dbl[])
      n81 = local write "vecEstufa"(w34) -> ()
      n82 = local write "ct_CEVAL"(w24) -> ()
      n83 = local write "increment"(w23) -> ()
      n84 = local write "Res_TempME"(w23) -> ()
      n85 = local write "bypass"(w23) -> ()
      n86 = local write "Skip"(w23) -> ()
      n87 = local write "teste"(w23) -> ()
      n88 = local write "reset"(w23) -> ()
      n89 = local write "ct_TempME"(w24) -> ()
      n90 = Initialize Array(-999.0 ("element"), 3 ("dimension size")) -> (w32:dbl[])
      n91 = local write "vec_CEVAL"(w32) -> ()
      n92 = Initialize Array(-999.0 ("element"), 3 ("dimension size")) -> (w27:dbl[])
      n93 = local write "vecTempME"(w27) -> ()
      n94 = disable-structure shown="Disabled" {
        disable-tunnel: [w84 _] -> w69
        frame Disabled {
          n95 = call "name_file.vi"("Identifier"="Logfile_6812B") -> ("appended path"=w84:path)  [unwired: 2 in]
        }
        frame Enabled {
        }
      }
      n96 = disable-structure shown="Enabled" {
        disable-tunnel: [w104 _] -> w56
        frame Disabled {
          n97 = call "name_file.vi"("Identifier"="Logfile_EEC") -> ("appended path"=w104:path)  [unwired: 2 in]
        }
        frame Enabled {
        }
      }
      n98 = call "name_file.vi"("Identifier"="Logfile_ETME") -> ("appended path"=w71:path)  [unwired: 2 in]
      n99 = call <instrlib>:"Initialize.vi"("VISA Resource Name"=refnum<visa-resource-name> "Agilent" ("VISA AGILENT")) -> ("VISA Resource Name Out"=w81:refnum<visa-resource-name>)  [unwired: 13 in, 1 out]
      n100 = call "name_file.vi"("Identifier"="Logfile_Watt") -> ("appended path"=w77:path)  [unwired: 2 in]
      n101 = call "name_file.vi"("Identifier"="Logfile_Estufa") -> ("appended path"=w80:path)  [unwired: 2 in]
      n102 = call "name_file.vi"("Identifier"="Logfile_Freio") -> ("appended path"=w75:path)  [unwired: 2 in]
      n103 = call "name_file.vi"("Identifier"="Logfile_Dina") -> ("appended path"=w64:path)  [unwired: 2 in]
      n104 = call "name_file.vi"("Identifier"="Logfile_TPs") -> ("appended path"=w73:path)  [unwired: 2 in]
      n105 = local write "STOP"(FALSE ("STOP")) -> ()
      n106 = call "name_file.vi"("Identifier"="Logfile_ETMI") -> ("appended path"=w38:path)  [unwired: 2 in]
      "PT100_CH4" <- w65
      "PT100_CH9" <- w65
      "Time" <- w65
      "Duty Cycle" <- sgl 0.01 ("Duty Cycle")
      "PV" <- w22
      "t" <- w22
      "Chart_tensao" <- T4 {"V(A)"=0.0, "V(B)"=0.0, "V(E)"=0.0, "V(E) 2"=0.0} ("Chart_tensao")
      "TP 1" <- w65
      "TP 2" <- w65
      "TP 3" <- w65
      "TP 5" <- w65
      "TP 6" <- w65
      "TP 7" <- w65
      "TP 8" <- w65
      "TP 10" <- w65
      "TP 11" <- w65
      "TP 12" <- w65
      "TP 13" <- w65
      "TP 15" <- w65
      "PV_MIC" <- w22
      "error out (6812B)" <- errorcluster {"status"=FALSE, "code"=0, "source"=""} ("error out")
      "ACP_CUR" <- T16 {"Peak Current"=0.0, "AC RMS Current"=0.0} ("ACP_CUR")
      "ACP_PWR" <- T17 {"Reactive Power"=0.0, "Apparent Power"=0.0} ("ACP_PWR")
      "volt_cluster" <- T4 {"V(A)"=0.0, "V(B)"=0.0, "V(E)"=0.0, "V(E) 2"=0.0} ("volt_cluster")
      "cur_cluster" <- T4 {"V(A)"=0.0, "V(B)"=0.0, "V(E)"=0.0, "V(E) 2"=0.0} ("cur_cluster")
      "pwr_cluster" <- T6 {"PC(A)"=0.0, "PC(B)"=0.0, "PC(T)"=0.0, "PL(A)"=0.0, "PL(B)"=0.0, "PL(T)"=0.0, "PC(E)"=0.0, "PL(E)"=0.0, "PL(E) 2"=0.0} ("pwr_cluster")
      "Chart_power" <- T6 {"PC(A)"=0.0, "PC(B)"=0.0, "PC(T)"=0.0, "PL(A)"=0.0, "PL(B)"=0.0, "PL(T)"=0.0, "PC(E)"=0.0, "PL(E)"=0.0, "PL(E) 2"=0.0} ("Chart_power")
      "Chart_cur" <- T5 {"I(A)"=0.0, "I(B)"=0.0, "I(E)"=0.0, "I(E) 2"=0.0} ("Chart_cur")
      "Chart_velo" <- cluster{"V(A)":dbl, "V(B)":dbl} {"V(A)"=0.0, "V(B)"=0.0} ("Chart_velo")
      "ACP_VOLT" <- cluster{"Peak Current":dbl} {"Peak Current"=0.0} ("ACP_VOLT")
      "EEC_VOLT" <- cluster{"Peak Current":dbl} {"Peak Current"=0.0} ("EEC_VOLT")
      "EEC_CURR" <- cluster{"Peak Current":dbl} {"Peak Current"=0.0} ("EEC_CURR")
      "EEC_PWR" <- cluster{"Peak Current":dbl} {"Peak Current"=0.0} ("EEC_PWR")
      "PW MP ok" <- w23
      "STEADY?" <- w23
      "STEADY MF?" <- w23
      "Final Ensaio" <- w23
      "LIM SS" <- w23
      "LIM SS MF" <- w23
      "Continue" <- w23
      "PV_MI" <- w22
      "CP EV ok" <- w23
      "ss_ceval" <- FALSE ("STEADY_CEVAL")
      "MV_ME" <- w22
      "MV_C1" <- w22
      "MV_L1" <- w22
      "MV_C5" <- w22
      "MV_MIC" <- w22
      "GME_C1" <- w21
      "Graf_MV_C1" <- w20
      "GME_L1" <- w21
      "GME_C5" <- w21
      "GME_MIC" <- w21
      "Graf_MV_L1" <- w20
      "Graf_MV_C5" <- w20
      "Graf_MV_MIC" <- w20
      "SPs_Filtro" <- T1 {"SP_F"=0.0, "SP_F"=0.0, "SP_F"=0.0, "SP_F"=0.0} ("SPs_Filtro")
    }
    frame #1 {
      # "Temporizador"
      n107 = disable-structure shown="Disabled" {
        disable-tunnel: w296 -> [w330 _]
        frame Disabled {
          n108 = call-poly <vilib>:"Write Delimited Spreadsheet.vi"("file path (dialog if empty)"=w330, "1D data"=string[] ["t", "PT[W]", "FP", "IP[A]", "IRMS[A]", "VRMS[V]", "", "", "", "", "", "", ""] ("appended array"), "append to file? (new file:F)"=TRUE, "transpose? (no:F)"=FALSE) -> ("new file path (Not A Path if cancelled)"=w326:path)  [unwired: 10 in, 1 out]
          n109 = while {
            tunnel: w326 -> [w358]
            stop <- w352 stop-if-true
            # "Fator de Potencia"
            # "Tensão AC RMS"
            # "Corrente AC + DC RMS"
            # "Corrente de Pico"
            # "Potência Total"
            # "tempo(s):"
            # "Gerando log das Medidas Elétricas da fonte 6812B"
            n110 = local read "VolMeas"() -> (w347:cluster{"AC + DC RMS Voltage":dbl})
            n111 = local read "PwrMeas"() -> (w344:cluster{"Total Power":dbl, "Power Factor":dbl})
            n112 = local read "CurMeas"() -> (w348:T18)
            n113 = Wait (ms)(milliseconds to wait=u32 25000) -> ()  [unwired: 1 out]
            n114 = Unbundle(w347) -> ("AC + DC RMS Voltage"=w332:dbl)
            n115 = Unbundle(w344) -> ("Total Power"=w338:dbl, "Power Factor"=w337:dbl)
            n116 = Unbundle(w348) -> ("Peak Current"=w335:dbl, "AC + DC RMS Cur"=w334:dbl)
            n117 = Bundle("Total Power"=w338, "Power Factor"=w337) -> (w336:cluster{"Total Power":dbl, "Power Factor":dbl})  [unwired: 1 in]
            n118 = Bundle("AC + DC RMS Voltage"=w332) -> (w331:cluster{"AC + DC RMS Voltage":dbl})  [unwired: 1 in]
            n119 = Bundle("Peak Current"=w335, "AC + DC RMS Cur"=w334) -> (w333:T18)  [unwired: 1 in]
            n120 = local read "t"() -> (w355:dbl)
            n121 = local write "ACP_VOLT"(w331) -> ()
            n122 = local write "ACP_PWR"(w336) -> ()
            n123 = local write "ACP_CUR"(w333) -> ()
            n124 = Number To Exponential String(number=w335, precision (6)=i16 3) -> (E-format string=w341:string)  [unwired: 2 in]
            n125 = Number To Exponential String(number=w334, precision (6)=i16 3) -> (E-format string=w340:string)  [unwired: 2 in]
            n126 = Number To Exponential String(number=w332, precision (6)=i16 3) -> (E-format string=w339:string)  [unwired: 2 in]
            n127 = Number To Exponential String(number=w338, precision (6)=i16 3) -> (E-format string=w345:string)  [unwired: 2 in]
            n128 = Number To Exponential String(number=w337, precision (6)=i16 3) -> (E-format string=w342:string)  [unwired: 2 in]
            n129 = Number To Fractional String(number=w355, precision (6)=i16 3) -> (F-format string=w354:string)  [unwired: 2 in]
            n130 = Build Array(w354, w345, w342, w341, w340, w339) -> (w353:string[])
            n131 = local read "STOP"() -> (w352:bool)
            n132 = call-poly <vilib>:"Write Delimited Spreadsheet.vi"("file path (dialog if empty)"=w358, "1D data"=w353, "append to file? (new file:F)"=TRUE, "transpose? (no:F)"=FALSE) -> ()  [unwired: 10 in, 2 out]
          }
        }
        frame Enabled {
        }
      }
      n133 = while {
        tunnel: w271 -> [w609]
        tunnel: w270 -> [w608]
        stop <- w611 stop-if-true
        n134 = local write "VISA  name (6812B)"(w608) -> ()
        n135 = local write "error out (6812B)"(w609) -> ()
        n136 = local read "STOP"() -> (w611:bool)
        n137 = Wait (ms)(milliseconds to wait=u32 1000) -> ()  [unwired: 1 out]
        n138 = disable-structure shown="Disabled" {
          frame Disabled {
            n139 = call "measPwrCur.vi"() -> ("VolMeas"=w613:cluster{"AC + DC RMS Voltage":dbl}, "CurMeas"=w614:T24, "PwrMeas"=w612:cluster{"Total Power":dbl, "Power Factor":dbl})  [unwired: 4 in, 2 out]
            n140 = local write "PwrMeas"(w612) -> ()
            n141 = local write "CurMeas"(w614) -> ()
            n142 = local write "VolMeas"(w613) -> ()
          }
          frame Enabled {
          }
        }
      }
      n143 = disable-structure shown="Disabled" {
        frame Disabled {
          n144 = call <instrlib>:"Close.vi"() -> ()  [unwired: 11 in, 1 out]
        }
        frame Enabled {
        }
      }
      n145 = disable-structure shown="Disabled" {
        disable-tunnel: w290 -> [w1095 _]
        disable-tunnel: w289 -> [w1094 _]
        frame Disabled {
          n146 = while {
            tunnel: w1095 -> [w1111]
            tunnel: w1094 -> [w1110]
            tunnel: [w1109] -> w1093
            tunnel: [w1099] -> w1092
            stop <- w1108 stop-if-true
            # "kW --> W"
            # "Faz as leituras/medições"
            n147 = local read "Configurações"() -> (w1107:T15)
            n148 = Unbundle By Name(w1107) -> ("Tensão (V)"=w1105:dbl)
            n149 = Wait Until Next ms Multiple(millisecond multiple=u32 1000 ("milliseconds to wait")) -> ()  [unwired: 1 out]
            n150 = call "Is Value Changed.vim"("value"=w1105) -> ("changed or first call?"=w1106:bool)
            n151 = case shown="False" w1106 {
              tunnel: [w1114 w1126] -> w1112
              tunnel: w1111 -> [w1118 w1123]
              tunnel: w1110 -> [w1117 w1122]
              tunnel: [w1115 w1125] -> w1109
              tunnel: [w1116 w1124] -> w1099
              tunnel: w1105 -> [_ w1121]
              frame False {
                n152 = call "Medicao(SubVI).vi"("error in (no error)"=w1117, "VISA Refnum in"=w1118) -> ("error out"=w1115:errorcluster, "All Measurements"=w1114:T25, "VISA Refnum out"=w1116:refnum<visa-resource-name>)  [unwired: 7 in]
              }
              frame True {
                # "8"
                n153 = call "Tensao_AC (SubVI).vi"("error in (no error)"=w1122, "Tensão (V)"=w1121, "VISA Refnum in"=w1123) -> ("error out"=w1119:errorcluster, "VISA Refnum out"=w1120:refnum<visa-resource-name>)  [unwired: 7 in]
                n154 = call "Medicao(SubVI).vi"("error in (no error)"=w1119, "VISA Refnum in"=w1120) -> ("error out"=w1125:errorcluster, "All Measurements"=w1126:T25, "VISA Refnum out"=w1124:refnum<visa-resource-name>)  [unwired: 7 in]
              }
            }
            n155 = Unbundle By Name(w1112) -> ("Frequency"=w1104:dbl, "AC Voltage"=w1103:dbl, "Current"=w1102:dbl, "Power"=w1098:dbl, "Power Factor"=w1101:dbl)
            n156 = Multiply(x=w1098, y=1000.0) -> (x*y=w1096:dbl)
            n157 = Bundle("Frequency"=w1104, "AC Voltage"=w1103, "Current"=w1102, w1096, "Power Factor"=w1101) -> (→"EEC_OUT":T26)  [unwired: 1 in]
            n158 = local read "STOP"() -> (w1108:bool)
          }
          n159 = VISA Close(VISA resource name=w1092, error in (no error)=w1093) -> ()  [unwired: 1 out]
        }
        frame Enabled {
        }
      }
      n160 = disable-structure shown="Disabled" {
        disable-tunnel: w288 -> [w1060 _]
        frame Disabled {
          n161 = call-poly <vilib>:"Write Delimited Spreadsheet.vi"("file path (dialog if empty)"=w1060, "1D data"=string[] ["t", "FREQ[Hz]", "VAC[V]", "IOUT[A]", "VRMS[V]", "POUT[W]", "FP", "", "", "", "", "", ""] ("appended array"), "append to file? (new file:F)"=TRUE, "transpose? (no:F)"=FALSE) -> ("new file path (Not A Path if cancelled)"=w1059:path)  [unwired: 10 in, 1 out]
          n162 = while {
            tunnel: w1059 -> [w1070]
            stop <- w1091 stop-if-true
            # "Fator de Potência"
            # "Potência(W):"
            # "Corrente (A)"
            # "Tensão AC (V):"
            # "Frequencia(Hz):"
            # "tempo(s):"
            n163 = local read "EEC_OUT"() -> (w1090:T20)
            n164 = Unbundle By Name(w1090) -> ("Frequency"=w1081:dbl, "AC Voltage"=w1068:dbl, "Current"=w1067:dbl, "Power"=w1064:dbl, "Power Factor"=w1080:dbl)
            n165 = Wait (ms)(milliseconds to wait=u32 1000) -> ()  [unwired: 1 out]
            n166 = Bundle("Power"=w1064) -> (w1065:cluster{"Power":dbl})  [unwired: 1 in]
            n167 = Bundle("AC Voltage"=w1068) -> (w1069:cluster{"AC Voltage":dbl})  [unwired: 1 in]
            n168 = Bundle("Current"=w1067) -> (w1066:cluster{"Current":dbl})  [unwired: 1 in]
            n169 = local write "EEC_PWR"(w1065) -> ()
            n170 = local write "EEC_CURR"(w1066) -> ()
            n171 = local write "EEC_VOLT"(w1069) -> ()
            n172 = local read "t"() -> (w1087:dbl)
            n173 = Number To Fractional String(number=w1087, precision (6)=i16 3) -> (F-format string=w1079:string)  [unwired: 2 in]
            n174 = Number To Fractional String(number=w1081, precision (6)=i16 3) -> (F-format string=w1078:string)  [unwired: 2 in]
            n175 = Number To Fractional String(number=w1068, precision (6)=i16 3) -> (F-format string=w1077:string)  [unwired: 2 in]
            n176 = Number To Fractional String(number=w1067, precision (6)=i16 3) -> (F-format string=w1076:string)  [unwired: 2 in]
            n177 = Number To Fractional String(number=w1064, precision (6)=i16 3) -> (F-format string=w1075:string)  [unwired: 2 in]
            n178 = Number To Fractional String(number=w1080, precision (6)=i16 3) -> (F-format string=w1074:string)  [unwired: 2 in]
            n179 = local read "STOP"() -> (w1091:bool)
            n180 = Build Array(w1079, w1078, w1077, w1076, w1075, w1074) -> (w1071:string[])
            n181 = call-poly <vilib>:"Write Delimited Spreadsheet.vi"("file path (dialog if empty)"=w1070, "1D data"=w1071, "append to file? (new file:F)"=TRUE, "transpose? (no:F)"=FALSE) -> ()  [unwired: 10 in, 2 out]
          }
        }
        frame Enabled {
        }
      }
      n182 = while {
        shift-right: [w617] -> _
        shift-left: T11."Read power" ("Message") -> [w618]
        stop <- w616 stop-if-true
        # "Loop para adquirir as medidas do inversor (tensao barramento, potencia entrada e velocidade real)"
        n183 = case shown="\"Read power\"" w618 {
          tunnel: [T11."Read bus voltage" ("Message") T11."Read real speed" ("Message") T11."Read operation status" ("Message") T11."Read power" ("Message")] -> w617
          frame "Read power" {
            w622 = 0 ("offset")
            # "Manda msg para ler valor da potencia do inversor"
            n184 = local read "Parâmetros serial"() -> (w624:T10)
            n185 = Wait (ms)(milliseconds to wait=u32 10) -> ()  [unwired: 1 out]
            n186 = call "Serial_control.vi"("Message"=T11."Read power", "Função"=T21."Send Static Message", "comm cluster"=w624) -> ("translated message"=w625:string)  [unwired: 2 in, 3 out]
            n187 = local write "Tradução"(w625) -> ()
            n188 = Decimal String To Number(string=w625, offset=w622, default (0L)=w622) -> (number=w626:i32)  [unwired: 1 out]
            n189 = local write "Pinv"(w626) -> ()
          }
          frame "Read bus voltage" {
            w631 = 0 ("offset")
            # "Manda msg para ler valor do BUS DC"
            n190 = local read "Parâmetros serial"() -> (w632:T10)
            n191 = Wait (ms)(milliseconds to wait=u32 10) -> ()  [unwired: 1 out]
            n192 = call "Serial_control.vi"("Message"=T11."Read bus voltage", "Função"=T21."Send Static Message", "comm cluster"=w632) -> ("translated message"=w633:string)  [unwired: 2 in, 3 out]
            n193 = local write "Tradução"(w633) -> ()
            n194 = Decimal String To Number(string=w633, offset=w631, default (0L)=w631) -> (number=w634:i32)  [unwired: 1 out]
            n195 = local write "DCBus"(w634) -> ()
          }
          frame "Read real speed" {
            w640 = 0 ("offset")
            # "Manda msg para ler valor de velocidade real"
            n196 = local read "Parâmetros serial"() -> (w641:T10)
            n197 = Wait (ms)(milliseconds to wait=u32 10) -> ()  [unwired: 1 out]
            n198 = call "Serial_control.vi"("Message"=T11."Read real speed", "Função"=T21."Send Static Message", "comm cluster"=w641) -> ("translated message"=w635:string)  [unwired: 2 in, 3 out]
            n199 = local write "Tradução"(w635) -> ()
            n200 = Decimal String To Number(string=w635, offset=w640, default (0L)=w640) -> (number=w642:i32)  [unwired: 1 out]
            n201 = local write "Vel Real"(w642) -> ()
          }
          frame "Read set speed", "Read operation status", "Read starting trials", "Read temperature".."Read PWM frequency" {
            n202 = Wait (ms)(milliseconds to wait=u32 1) -> ()  [unwired: 1 out]
          }
        }
        n203 = local read "STOP"() -> (w616:bool)
        n204 = Wait (ms)(milliseconds to wait=u32 1000) -> ()  [unwired: 1 out]
      }
      n205 = call-poly <vilib>:"Write Delimited Spreadsheet.vi"("file path (dialog if empty)"=w298, "1D data"=string[] ["t", "SP_C1 [ºC]", "MV_C1 [W]", "SP_L1 [ºC]", "MV_L1 [W]", "SP_C5 [ºC]", "MV_C5 [W]", "SP_MIC [ºC]", "MV_MIC [W]", "MV_ME [W]", "SPF_C1[°C]", "SPF_L1[°C]", "SPF_C5[°C]", "SPF_MIC[°C]"] ("appended array"), "append to file? (new file:F)"=TRUE, "transpose? (no:F)"=FALSE) -> ("new file path (Not A Path if cancelled)"=w297:path)  [unwired: 10 in, 1 out]
      n206 = call-poly <vilib>:"Write Delimited Spreadsheet.vi"("file path (dialog if empty)"=w321, "1D data"=string[] ["t", "PV [ºC]", "SP [ºC]", "MV[%] "] ("appended array"), "append to file? (new file:F)"=TRUE, "transpose? (no:F)"=FALSE) -> ("new file path (Not A Path if cancelled)"=w322:path)  [unwired: 10 in, 1 out]
      n207 = call-poly <vilib>:"Write Delimited Spreadsheet.vi"("file path (dialog if empty)"=w320, "1D data"=string[] ["t", "PL(A)", "PL(B)", "PL(T)", "PL(E)", "V(A)", "V(B)", "V(E)", "I(A)", "I(B)", "I(E)"] ("appended array"), "append to file? (new file:F)"=TRUE, "transpose? (no:F)"=FALSE) -> ("new file path (Not A Path if cancelled)"=w316:path)  [unwired: 10 in, 1 out]
      n208 = call-poly <vilib>:"Write Delimited Spreadsheet.vi"("file path (dialog if empty)"=w315, "1D data"=string[] ["t", "IF", "IR", "VF", "VR", "VelSP", "VelRE", "DCbus", "PINV"] ("appended array"), "append to file? (new file:F)"=TRUE, "transpose? (no:F)"=FALSE) -> ("new file path (Not A Path if cancelled)"=w311:path)  [unwired: 10 in, 1 out]
      n209 = call-poly <vilib>:"Write Delimited Spreadsheet.vi"("file path (dialog if empty)"=w293, "1D data"=string[] ["t", "T_FR", "T_B1", "T_B2", "T_E2", "T_E1", "T_AMB"] ("appended array"), "append to file? (new file:F)"=TRUE, "transpose? (no:F)"=FALSE) -> ("new file path (Not A Path if cancelled)"=w291:path)  [unwired: 10 in, 1 out]
      n210 = call-poly <vilib>:"Write Delimited Spreadsheet.vi"("file path (dialog if empty)"=w306, "1D data"=string[] ["t", "TP1", "TP2", "TP3", "TP5", "TP6", "TP7", "TP8", "TP10", "TP11", "TP12", "TP13", "TP15"] ("appended array"), "append to file? (new file:F)"=TRUE, "transpose? (no:F)"=FALSE) -> ("new file path (Not A Path if cancelled)"=w305:path)  [unwired: 10 in, 1 out]
      n211 = call-poly <vilib>:"Write Delimited Spreadsheet.vi"("file path (dialog if empty)"=w286, "1D data"=string[] ["t", "PV [W]", "SP [W]", "MV[I]"] ("appended array"), "append to file? (new file:F)"=TRUE, "transpose? (no:F)"=FALSE) -> ("new file path (Not A Path if cancelled)"=w282:path)  [unwired: 10 in, 1 out]
      n212 = call <vilib>:"High Resolution Relative Seconds.vi"() -> ("relative seconds"=w310:dbl)
      n213 = while {
        tunnel: w297 -> [w1276]
        stop <- w1265 stop-if-true
        # "SP filtrado PI-MIC"
        # "SP filtrado PI-C5"
        # "SP filtrado PI-L1"
        # "SP filtrado PI-C1"
        # "MV controlador override"
        # "Referencia do MIC"
        # "MV controlador de MIC"
        # "Referencia Cap C5"
        # "MV controlador de C5"
        # "Referencia ind L1"
        # "MV controlador de L1"
        # "tempo(s):"
        # "Referencia Cap C1"
        # "MV controlador de C1"
        # "Gerando log do Controle do Ensaio Térmico para Malha Externa"
        n214 = local read "Ts ME"() -> (w1230:dbl)
        n215 = local read "SPs_Filtro"() -> (w1239:T1)
        n216 = Multiply(x=w1230, y=u32 1000 ("milliseconds to wait")) -> (x*y=w1228:dbl)
        n217 = local read "MV_L1"() -> (w1264:dbl)
        n218 = local read "MV_MIC"() -> (w1256:dbl)
        n219 = local read "MV_C5"() -> (w1257:dbl)
        n220 = local read "SP_L1"() -> (w1262:dbl)
        n221 = local read "SP_MIC"() -> (w1254:dbl)
        n222 = local read "MV_C1"() -> (w1268:dbl)
        n223 = local read "SP_C5"() -> (w1259:dbl)
        n224 = local read "SP_C1"() -> (w1274:dbl)
        n225 = local read "MV_ME"() -> (w1251:sgl)
        n226 = Unbundle(w1239) -> ("SP_F"=w1238:dbl, "SP_F"=w1237:dbl, "SP_F"=w1236:dbl, "SP_F"=w1235:dbl)
        n227 = local read "t"() -> (w1272:dbl)
        n228 = Wait (ms)(milliseconds to wait=w1228) -> ()  [unwired: 1 out]
        n229 = Number To Fractional String(number=w1262, precision (6)=i16 3) -> (F-format string=w1250:string)  [unwired: 2 in]
        n230 = Number To Fractional String(number=w1264, precision (6)=i16 3) -> (F-format string=w1249:string)  [unwired: 2 in]
        n231 = Number To Fractional String(number=w1259, precision (6)=i16 3) -> (F-format string=w1248:string)  [unwired: 2 in]
        n232 = Number To Fractional String(number=w1257, precision (6)=i16 3) -> (F-format string=w1247:string)  [unwired: 2 in]
        n233 = Number To Fractional String(number=w1272, precision (6)=i16 3) -> (F-format string=w1271:string)  [unwired: 2 in]
        n234 = Number To Fractional String(number=w1274, precision (6)=i16 3) -> (F-format string=w1270:string)  [unwired: 2 in]
        n235 = Number To Fractional String(number=w1268, precision (6)=i16 3) -> (F-format string=w1266:string)  [unwired: 2 in]
        n236 = Number To Fractional String(number=w1254, precision (6)=i16 3) -> (F-format string=w1246:string)  [unwired: 2 in]
        n237 = Number To Fractional String(number=w1256, precision (6)=i16 3) -> (F-format string=w1245:string)  [unwired: 2 in]
        n238 = Number To Fractional String(number=w1251, precision (6)=i16 3) -> (F-format string=w1244:string)  [unwired: 2 in]
        n239 = Number To Fractional String(number=w1238, precision (6)=i16 3) -> (F-format string=w1234:string)  [unwired: 2 in]
        n240 = Number To Fractional String(number=w1237, precision (6)=i16 3) -> (F-format string=w1233:string)  [unwired: 2 in]
        n241 = Number To Fractional String(number=w1236, precision (6)=i16 3) -> (F-format string=w1232:string)  [unwired: 2 in]
        n242 = Number To Fractional String(number=w1235, precision (6)=i16 3) -> (F-format string=w1231:string)  [unwired: 2 in]
        n243 = Build Array(w1271, w1270, w1266, w1250, w1249, w1248, w1247, w1246, w1245, w1244, w1234, w1233, w1232, w1231) -> (w1267:string[])
        n244 = local read "STOP"() -> (w1265:bool)
        n245 = call-poly <vilib>:"Write Delimited Spreadsheet.vi"("file path (dialog if empty)"=w1276, "1D data"=w1267, "append to file? (new file:F)"=TRUE, "transpose? (no:F)"=FALSE) -> ()  [unwired: 10 in, 2 out]
      }
      n246 = while {
        tunnel: w282 -> [w868]
        stop <- w853 stop-if-true
        # "tempo(s):"
        # "Saída (PV):"
        # "Referencia (SP):"
        # "sinal de controle (mv):"
        # "Gerando log do Controle do Ensaio Térmico para Malha Interna"
        n247 = local read "MV_MI"() -> (w864:dbl)
        n248 = local read "SP_Pwr"() -> (w857:i32)
        n249 = local read "PV_MI"() -> (w863:dbl)
        n250 = local read "Time"() -> (w861:dbl)
        n251 = Number To Exponential String(number=w864, precision (6)=i16 6) -> (E-format string=w866:string)  [unwired: 2 in]
        n252 = Number To Fractional String(number=w861, precision (6)=i16 6) -> (F-format string=w860:string)  [unwired: 2 in]
        n253 = Number To Fractional String(number=w863, precision (6)=i16 6) -> (F-format string=w859:string)  [unwired: 2 in]
        n254 = Number To Fractional String(number=w857, precision (6)=i16 6) -> (F-format string=w855:string)  [unwired: 2 in]
        n255 = Build Array(w860, w859, w855, w866) -> (w856:string[])
        n256 = local read "STOP"() -> (w853:bool)
        n257 = call-poly <vilib>:"Write Delimited Spreadsheet.vi"("file path (dialog if empty)"=w868, "1D data"=w856, "append to file? (new file:F)"=TRUE, "transpose? (no:F)"=FALSE) -> ()  [unwired: 10 in, 2 out]
        n258 = Wait Until Next ms Multiple(millisecond multiple=u32 100 ("milliseconds to wait")) -> ()  [unwired: 1 out]
      }
      n259 = while {
        tunnel: w322 -> [w1582]
        stop <- w1567 stop-if-true
        # "tempo(s):"
        # "Saída (PV):"
        # "Referencia (SP):"
        # "sinal de controle (mv):"
        # "Gerando log do Controle de Temperatura da Estufa"
        n260 = local read "Duty Cycle"() -> (w1579:sgl)
        n261 = Wait (ms)(milliseconds to wait=u32 1000) -> ()  [unwired: 1 out]
        n262 = local read "SP:"() -> (w1572:dbl)
        n263 = local read "PV"() -> (w1578:dbl)
        n264 = local read "t"() -> (w1576:dbl)
        n265 = Number To Fractional String(number=w1576, precision (6)=i16 3) -> (F-format string=w1575:string)  [unwired: 2 in]
        n266 = Number To Fractional String(number=w1578, precision (6)=i16 3) -> (F-format string=w1574:string)  [unwired: 2 in]
        n267 = Number To Fractional String(number=w1572, precision (6)=i16 3) -> (F-format string=w1570:string)  [unwired: 2 in]
        n268 = Number To Exponential String(number=w1579, precision (6)=i16 3) -> (E-format string=w1580:string)  [unwired: 2 in]
        n269 = Build Array(w1575, w1574, w1570, w1580) -> (w1571:string[])
        n270 = local read "STOP"() -> (w1567:bool)
        n271 = call-poly <vilib>:"Write Delimited Spreadsheet.vi"("file path (dialog if empty)"=w1582, "1D data"=w1571, "append to file? (new file:F)"=TRUE, "transpose? (no:F)"=FALSE) -> ()  [unwired: 10 in, 2 out]
      }
      n272 = while {
        tunnel: w311 -> [w1457]
        tunnel: w310 -> [w1437]
        stop <- w1443 stop-if-true
        # "Potência medida pelo inversor:"
        # "Tensão de barramento do inversor:"
        # "Velocidade atual do motor:"
        # "SP de velocidade do motor:"
        # "era 200"
        # "Tensão do freio (SP) [V]:"
        # "tempo(s):"
        # "Corrente de saída da fonte [A]:"
        # "Corrente do freio (SP) [A]:"
        # "Tensão de saída da Fonte [V]"
        # "Gerando log dos valores de tensão e corrente enviados ao freio + velocidade lida pelo inversor"
        n273 = call <vilib>:"High Resolution Relative Seconds.vi"() -> ("relative seconds"=w1438:dbl)
        n274 = Subtract(x=w1438, y=w1437) -> (x-y=w1436:dbl)
        n275 = local write "t"(w1436) -> ()
        n276 = local read "Limite de corrente"() -> (w1446:dbl)
        n277 = local read "Velocidade (RPM)"() -> (w1431:u16)
        n278 = local read "Corrente de saída"() -> (w1452:dbl)
        n279 = local read "Limite de tensão"() -> (w1441:dbl)
        n280 = local read "Tensão de saída"() -> (w1453:dbl)
        n281 = local read "Vel Real"() -> (w1430:u16)
        n282 = local read "DCBus"() -> (w1427:u16)
        n283 = local read "Pinv"() -> (w1424:u16)
        n284 = Bundle("Velocidade (RPM)"=w1431, "Vel Real"=w1430) -> (w1429:cluster{"Velocidade (RPM)":u16, "Vel Real":u16})  [unwired: 1 in]
        n285 = local read "t"() -> (w1450:dbl)
        n286 = disable-structure shown="Disabled" {
          disable-tunnel: w1429 -> [w1460 _]
          frame Disabled {
            n287 = local write "Chart_velo"(w1460) -> ()
          }
          frame Enabled {
          }
        }
        n288 = Number To Fractional String(number=w1450, precision (6)=i16 3) -> (F-format string=w1449:string)  [unwired: 2 in]
        n289 = Number To Fractional String(number=w1452, precision (6)=i16 3) -> (F-format string=w1448:string)  [unwired: 2 in]
        n290 = Number To Fractional String(number=w1446, precision (6)=i16 3) -> (F-format string=w1444:string)  [unwired: 2 in]
        n291 = Number To Exponential String(number=w1453, precision (6)=i16 3) -> (E-format string=w1455:string)  [unwired: 2 in]
        n292 = Number To Exponential String(number=w1441, precision (6)=i16 3) -> (E-format string=w1439:string)  [unwired: 2 in]
        n293 = Number To Exponential String(number=w1431, precision (6)=i16 3) -> (E-format string=w1434:string)  [unwired: 2 in]
        n294 = Number To Exponential String(number=w1430, precision (6)=i16 3) -> (E-format string=w1432:string)  [unwired: 2 in]
        n295 = Number To Exponential String(number=w1427, precision (6)=i16 3) -> (E-format string=w1428:string)  [unwired: 2 in]
        n296 = Number To Exponential String(number=w1424, precision (6)=i16 3) -> (E-format string=w1423:string)  [unwired: 2 in]
        n297 = Build Array(w1449, w1448, w1444, w1455, w1439, w1434, w1432, w1428, w1423) -> (w1445:string[])
        n298 = call-poly <vilib>:"Write Delimited Spreadsheet.vi"("file path (dialog if empty)"=w1457, "1D data"=w1445, "append to file? (new file:F)"=TRUE, "transpose? (no:F)"=FALSE) -> ()  [unwired: 10 in, 2 out]
        n299 = local read "STOP"() -> (w1443:bool)
        n300 = Wait (ms)(milliseconds to wait=u32 1000) -> ()  [unwired: 1 out]
      }
      n301 = while {
        tunnel: w305 -> [w1420]
        stop <- w1407 stop-if-true
        # "Termopar Dissipador"
        # "Termopar uC IC601"
        # "Termopar Cap 504"
        # "Termopar Cap C112"
        # "Termopar Indutor L100"
        # "Termopar  IC100"
        # "Termopar Conector"
        # "Termopar Fusivel"
        # "Termopar Cap C006"
        # "tempo(s):"
        # "Termopar Cap C011"
        # "Termopar Cap C009"
        # "Termopar Choke L001"
        # "Gerando log das Temperaturas dos Termopares"
        n302 = local read "TP 3"() -> (w1417:dbl)
        n303 = local read "TP 5"() -> (w1404:dbl)
        n304 = local read "TP 6"() -> (w1403:dbl)
        n305 = local read "TP 7"() -> (w1400:dbl)
        n306 = local read "TP 8"() -> (w1399:dbl)
        n307 = local read "TP 10"() -> (w1396:dbl)
        n308 = local read "TP 11"() -> (w1395:dbl)
        n309 = local read "TP 12"() -> (w1392:dbl)
        n310 = local read "TP 13"() -> (w1391:dbl)
        n311 = local read "TP 15"() -> (w1389:dbl)
        n312 = local read "TP 2"() -> (w1411:dbl)
        n313 = local read "TP 1"() -> (w1406:dbl)
        n314 = local read "t"() -> (w1415:dbl)
        n315 = Number To Fractional String(number=w1415, precision (6)=i16 3) -> (F-format string=w1414:string)  [unwired: 2 in]
        n316 = Number To Fractional String(number=w1406, precision (6)=i16 3) -> (F-format string=w1413:string)  [unwired: 2 in]
        n317 = Number To Fractional String(number=w1411, precision (6)=i16 3) -> (F-format string=w1409:string)  [unwired: 2 in]
        n318 = Number To Exponential String(number=w1417, precision (6)=i16 3) -> (E-format string=w1418:string)  [unwired: 2 in]
        n319 = Number To Exponential String(number=w1404, precision (6)=i16 3) -> (E-format string=w1388:string)  [unwired: 2 in]
        n320 = Number To Exponential String(number=w1403, precision (6)=i16 3) -> (E-format string=w1387:string)  [unwired: 2 in]
        n321 = Number To Exponential String(number=w1400, precision (6)=i16 3) -> (E-format string=w1386:string)  [unwired: 2 in]
        n322 = Number To Exponential String(number=w1399, precision (6)=i16 3) -> (E-format string=w1385:string)  [unwired: 2 in]
        n323 = Number To Exponential String(number=w1396, precision (6)=i16 3) -> (E-format string=w1384:string)  [unwired: 2 in]
        n324 = Number To Exponential String(number=w1395, precision (6)=i16 3) -> (E-format string=w1383:string)  [unwired: 2 in]
        n325 = Number To Exponential String(number=w1392, precision (6)=i16 3) -> (E-format string=w1382:string)  [unwired: 2 in]
        n326 = Number To Exponential String(number=w1391, precision (6)=i16 3) -> (E-format string=w1381:string)  [unwired: 2 in]
        n327 = Number To Exponential String(number=w1389, precision (6)=i16 3) -> (E-format string=w1380:string)  [unwired: 2 in]
        n328 = Build Array(w1414, w1413, w1409, w1418, w1388, w1387, w1386, w1385, w1384, w1383, w1382, w1381, w1380) -> (w1410:string[])
        n329 = local read "Ts ME"() -> (w1377:dbl)
        n330 = call-poly <vilib>:"Write Delimited Spreadsheet.vi"("file path (dialog if empty)"=w1420, "1D data"=w1410, "append to file? (new file:F)"=TRUE, "transpose? (no:F)"=FALSE) -> ()  [unwired: 10 in, 2 out]
        n331 = local read "STOP"() -> (w1407:bool)
        n332 = Multiply(x=w1377, y=u32 1000 ("milliseconds to wait")) -> (x*y=w1376:dbl)
        n333 = Wait (ms)(milliseconds to wait=w1376) -> ()  [unwired: 1 out]
      }
      n334 = while {
        tunnel: w316 -> [w1500]
        stop <- w1489 stop-if-true
        # "Corrente IB:"
        # "Corrente entrada do inversor:"
        # "Corrente IA:"
        # "Tensao entrada do inversor:"
        # "Tensao VCB:"
        # "Tensao VAB:"
        # "Pot. lida na entrada do inversor:"
        # "Pot. lida total"
        # "tempo(s):"
        # "Pot. lida na fase A:"
        # "Pot. lida na fase B:"
        # "Gerando log das potências medidas  do IF feitas pelo  Wattímetro"
        n335 = local read "pwr_cluster"() -> (w1483:T7)
        n336 = local read "volt_cluster"() -> (w1482:T9)
        n337 = local read "cur_cluster"() -> (w1481:T8)
        n338 = Unbundle(w1483) -> ("PL(A)"=w1480:dbl, "PL(B)"=w1472:dbl, "PL(T)"=w1479:dbl, "PL(E) - 6812B"=w1478:dbl)  [unwired: 5 out]
        n339 = Unbundle(w1482) -> ("V(A)"=w1467:dbl, "V(B)"=w1471:dbl, "V(E) - 6812B"=w1461:dbl)  [unwired: 1 out]
        n340 = Unbundle(w1481) -> ("I(A)"=w1470:dbl, "I(B)"=w1469:dbl, "I(E) - 6812B"=w1468:dbl)  [unwired: 1 out]
        n341 = local read "t"() -> (w1495:dbl)
        n342 = Number To Fractional String(number=w1495, precision (6)=i16 3) -> (F-format string=w1494:string)  [unwired: 2 in]
        n343 = Number To Fractional String(number=w1480, precision (6)=i16 3) -> (F-format string=w1493:string)  [unwired: 2 in]
        n344 = Number To Fractional String(number=w1472, precision (6)=i16 3) -> (F-format string=w1490:string)  [unwired: 2 in]
        n345 = Number To Exponential String(number=w1479, precision (6)=i16 3) -> (E-format string=w1498:string)  [unwired: 2 in]
        n346 = Number To Exponential String(number=w1478, precision (6)=i16 3) -> (E-format string=w1487:string)  [unwired: 2 in]
        n347 = Number To Exponential String(number=w1467, precision (6)=i16 3) -> (E-format string=w1484:string)  [unwired: 2 in]
        n348 = Number To Exponential String(number=w1471, precision (6)=i16 3) -> (E-format string=w1466:string)  [unwired: 2 in]
        n349 = Number To Exponential String(number=w1461, precision (6)=i16 3) -> (E-format string=w1465:string)  [unwired: 2 in]
        n350 = Number To Exponential String(number=w1470, precision (6)=i16 3) -> (E-format string=w1464:string)  [unwired: 2 in]
        n351 = Number To Exponential String(number=w1469, precision (6)=i16 3) -> (E-format string=w1463:string)  [unwired: 2 in]
        n352 = Number To Exponential String(number=w1468, precision (6)=i16 3) -> (E-format string=w1462:string)  [unwired: 2 in]
        n353 = Build Array(w1494, w1493, w1490, w1498, w1487, w1484, w1466, w1465, w1464, w1463, w1462) -> (w1491:string[])
        n354 = local read "STOP"() -> (w1489:bool)
        n355 = call-poly <vilib>:"Write Delimited Spreadsheet.vi"("file path (dialog if empty)"=w1500, "1D data"=w1491, "append to file? (new file:F)"=TRUE, "transpose? (no:F)"=FALSE) -> ()  [unwired: 10 in, 2 out]
        n356 = Wait (ms)(milliseconds to wait=u32 1000) -> ()  [unwired: 1 out]
      }
      n357 = while {
        stop <- w1127 stop-if-true
        # "Aquisição - Wattímetro WT230"
        n358 = local read "Realiza medição WT230"() -> (w1128:bool)
        n359 = case shown="True" w1128 {
          frame False {
            n360 = Wait (ms)(milliseconds to wait=u32 100) -> ()  [unwired: 1 out]
          }
          frame True {
            n361 = flat-sequence {
              frame #0 {
                n362 = property on="Realiza medição WT230" class="Bool (strict)"("DisabledEnum"=T22."Disabled and Grayed Out" ("Disabled")) -> ()  [unwired: 2 in, 2 out]
              }
              frame #1 {
                w1133 = u16 0 items=["Normal", "Continuous"] ("Integ Mode (0: Normal)")
                w1134 = u32 0 ("Hour (0)")
                n363 = call <instrlib>:"Config Integration.vi"("VISA resource name"=refnum<visa-resource-name> "WT", "Integ Mode (0: Normal)"=w1133, "Hour (0)"=w1134, "Minute (0)"=w1134, "Second (0)"="Tempo de integração (s)") -> ("VISA resource name out"=w1136:refnum<visa-resource-name>, "error out"=w1135:errorcluster)  [unwired: 9 in]
                n364 = while {
                  shift-right: [w1140] -> _
                  shift-left: w1136 -> [w1138]
                  shift-right: [w1139] -> _
                  shift-left: w1135 -> [w1137]
                  stop <- w1141 stop-if-true
                  w1147 = u16 1 items=["Clear", "Normal", "Integrate"] ("Preset Pattern (0: Clear)")
                  n365 = local read "Medição contínua? WT230"() -> (w1143:bool)
                  n366 = call <instrlib>:"Config Measure Preset Normal.vi"("VISA resource name"=w1138, "Preset Pattern (0: Clear)"=w1147, "error in (no error)"=w1137) -> ("VISA resource name out"=w1149:refnum<visa-resource-name>, "error out"=w1148:errorcluster)  [unwired: 11 in]
                  n367 = local read "STOP"() -> (w1144:bool)
                  n368 = call <instrlib>:"Start Stop Integration.vi"("VISA resource name"=w1149, "Start/Stop (F: Stop)"=TRUE, "error in (no error)"=w1148) -> ("VISA resource name out"=w1152:refnum<visa-resource-name>, "error out"=w1151:errorcluster)  [unwired: 11 in]
                  n369 = Not(x=w1143) -> (.not. x?=w1142:bool)
                  n370 = Or(x=w1142, y=w1144) -> (x .or. y?=w1141:bool)
                  n371 = while {
                    shift-left: w1152 -> [w1195]
                    shift-right: [w1183] -> w1146
                    shift-left: w1151 -> [w1192]
                    shift-right: [w1181] -> w1145
                    stop <- w1191 continue-if-true
                    w1198 = u16 2  # Integration indicated bit
                    # "Incluindo medidas(V,I,P) de entrada no grafico e no display, pois os valores de V(E), I(E) e P(E) lidos pelo Wattimetro vem da fonte 6812B e não da EEC 6510 (que alimenta o inversor)"
                    # "era 200"
                    # "mudei de 500 pra 1000"
                    n372 = call <instrlib>:"Read Measure.vi"("VISA resource name"=w1195, "error in (no error)"=w1192) -> ("VISA resource name out"=w1194:refnum<visa-resource-name>, "Measure Value"=w1185:sgl[], "error out"=w1193:errorcluster)  [unwired: 10 in, 1 out]
                    n373 = call <instrlib>:"Query Condition Status.vi"("VISA resource name"=w1194, "error in (no error)"=w1193) -> ("VISA resource name out"=w1180:refnum<visa-resource-name>, "Condition"=w1196:u16, "error out"=w1179:errorcluster)  [unwired: 11 in]
                    n374 = And(x=w1196, y=w1198) -> (x .and. y?=w1197:u16)
                    n375 = Not Equal To 0?(x=w1197) -> (x != 0?=w1191:bool)
                    n376 = case shown="False" w1191 {
                      tunnel: [w1212 w1219] -> w1190
                      tunnel: [w1211 w1219] -> w1189
                      tunnel: [w1210 w1219] -> w1188
                      tunnel: [w1209 w1219] -> w1187
                      tunnel: [w1208 w1218] -> w1184
                      tunnel: [w1207 w1217] -> w1182
                      tunnel: w1180 -> [w1206 w1218]
                      tunnel: w1179 -> [w1205 w1217]
                      frame False {
                        w1213 = u16 2 items=["Clear", "Normal", "Integrate"] ("Preset Pattern (0: Clear)")
                        n377 = call <instrlib>:"Config Measure Preset Normal.vi"("VISA resource name"=w1206, "Preset Pattern (0: Clear)"=w1213, "error in (no error)"=w1205) -> ("VISA resource name out"=w1216:refnum<visa-resource-name>, "error out"=w1215:errorcluster)  [unwired: 11 in]
                        n378 = call <instrlib>:"Read Measure.vi"("VISA resource name"=w1216, "error in (no error)"=w1215) -> ("VISA resource name out"=w1208:refnum<visa-resource-name>, "Measure Value"=w1214:sgl[], "error out"=w1207:errorcluster)  [unwired: 10 in, 1 out]
                        n379 = call "integration_translator.vi"("Valores integração"=w1214) -> ("PI(E)"=w1209:sgl, "PI(T)"=w1210:sgl, "PI(B)"=w1211:sgl, "PI(A)"=w1212:sgl)  [unwired: 7 in]
                      }
                      frame True {
                        w1219 = nan
                      }
                    }
                    n380 = local read "EEC_OUT"() -> (w1158:T20)
                    n381 = call <vilib>:"High Resolution Relative Seconds.vi"() -> ("relative seconds"=w1186:dbl)
                    n382 = call "measurements_to_cluster.vi"("PI(E)"=w1187, "PI(T)"=w1188, "relative seconds"=w1186, "PI(B)"=w1189, "PI(A)"=w1190, "Measure Value"=w1185) -> ("watt cluster"=w1178:T27)  [unwired: 4 in, 1 out]
                    n383 = Unbundle By Name(w1158) -> ("AC Voltage"=w1157:dbl, "Current"=w1155:dbl, "Power"=w1154:dbl)  [unwired: 1 out]
                    n384 = stacked-sequence {
                      tunnel: w1184 -> [w1203]
                      tunnel: [w1203] -> w1183
                      tunnel: w1182 -> [w1202]
                      tunnel: [w1202] -> w1181
                      frame #0 {
                        w1204 = u32 100  # Interval
                        n385 = Wait (ms)(milliseconds to wait=w1204) -> ()  [unwired: 1 out]
                      }
                    }
                    n386 = Unbundle By Name(w1178) -> ("V(A)"=w1177:dbl, "V(B)"=w1176:dbl, "V(E)"=w1175:dbl, "I(A)"=w1174:dbl, "I(B)"=w1173:dbl, "I(E)"=w1172:dbl, "PC(A)"=w1167:dbl, "PC(B)"=w1165:dbl, "PC(T)"=w1171:dbl, "PL(A)"=w1170:dbl, "PL(B)"=w1169:dbl, "PL(T)"=w1153:dbl, "PC(E)"=w1163:dbl, "PL(E)"=w1161:dbl)
                    n387 = Bundle("V(A)"=w1177, "V(B)"=w1176, "V(E)"=w1175, "AC Voltage"=w1157) -> (w1156:T28)  [unwired: 1 in]
                    n388 = Bundle("I(A)"=w1174, "I(B)"=w1173, "I(E)"=w1172, "Current"=w1155) -> (w1160:T29)  [unwired: 1 in]
                    n389 = call "filter.vi"("input"=w1167) -> ("output"=w1166:dbl)  [unwired: 10 in]
                    n390 = call "filter.vi"("input"=w1165) -> ("output"=w1164:dbl)  [unwired: 10 in]
                    n391 = call "filter.vi"("input"=w1171) -> ("output"=w1168:dbl)  [unwired: 10 in]
                    n392 = call "filter.vi"("input"=w1163) -> ("output"=w1162:dbl)  [unwired: 10 in]
                    n393 = local write "PV_MI"(w1153) -> ()
                    n394 = Bundle("output"=w1166, "output"=w1164, "output"=w1168, "PL(A)"=w1170, "PL(B)"=w1169, "PL(T)"=w1153, "output"=w1162, "PL(E)"=w1161, "Power"=w1154) -> (w1159:T30)  [unwired: 1 in]
                    n395 = disable-structure shown="Disabled" {
                      disable-tunnel: w1156 -> [w1201 _]
                      frame Disabled {
                        n396 = local write "Chart_tensao"(w1201) -> ()
                      }
                      frame Enabled {
                      }
                    }
                    n397 = disable-structure shown="Disabled" {
                      disable-tunnel: w1160 -> [w1200 _]
                      frame Disabled {
                        n398 = local write "Chart_cur"(w1200) -> ()
                      }
                      frame Enabled {
                      }
                    }
                    n399 = disable-structure shown="Disabled" {
                      disable-tunnel: w1159 -> [w1199 _]
                      frame Disabled {
                        n400 = local write "Chart_power"(w1199) -> ()
                      }
                      frame Enabled {
                      }
                    }
                    n401 = local write "volt_cluster"(w1156) -> ()
                    n402 = local write "cur_cluster"(w1160) -> ()
                    n403 = local write "pwr_cluster"(w1159) -> ()
                  }
                  n404 = call <instrlib>:"Reset Integration.vi"("VISA resource name"=w1146, "error in (no error)"=w1145) -> ("VISA resource name out"=w1140:refnum<visa-resource-name>, "error out"=w1139:errorcluster)  [unwired: 12 in]
                }
              }
              frame #2 {
                n405 = local write "Realiza medição WT230"(FALSE ("Realiza medição")) -> ()
                n406 = property on="Realiza medição WT230" class="Bool (strict)"("DisabledEnum"=T22."Enabled" ("Disabled")) -> ()  [unwired: 2 in, 2 out]
              }
            }
          }
        }
        n407 = local read "STOP"() -> (w1127:bool)
      }
      n408 = local read "vecEstufa"() -> (w281:dbl[])
      n409 = Obtain Notifier(notification data type=FALSE) -> (notifier out=w277:refnum<notifier>, error out=w278:errorcluster)  [unwired: 3 in, 1 out]
      n410 = Tick Count (ms)() -> (millisecond timer value=w287:u32)
      n411 = while {
        tunnel: w277 -> [w693]
        stop <- w692 stop-if-true
        n412 = Wait on Notification(notifier=w693) -> (notification=w691:bool, error out=w692:errorcluster)  [unwired: 3 in, 2 out]
        n413 = case shown="True" w691 {
          frame False {
            n414 = local write "LIM SS"(FALSE ("Boolean 2")) -> ()
          }
          frame True {
            n415 = local write "LIM SS"(TRUE ("Boolean 2")) -> ()
          }
        }
      }
      n416 = while {
        shift-right: [w931] -> _
        shift-left: w281 -> [w941]
        shift-right: [w935] -> _
        shift-left: w287 -> [w934]
        tunnel: w278 -> [w924]
        tunnel: w277 -> [w923]
        tunnel: [w922] -> w276
        tunnel: [w921] -> w275
        stop <- w929 stop-if-true
        # "ms"
        # "ms"
        # "s"
        # "Verifica se a temperatura da estufa atingiu o regime permanente"
        n417 = local read "TBR (min)"() -> (w927:u32)
        n418 = Tick Count (ms)() -> (millisecond timer value=w937:u32)
        n419 = local read "reset"() -> (w925:bool)
        n420 = Multiply(x=w927, y=u32 60) -> (x*y=w932:u32)
        n421 = Subtract(x=w937, y=w934) -> (x-y=w938:u32)
        n422 = Multiply(x=w932, y=u32 1000) -> (x*y=w940:u32)
        n423 = Greater Or Equal?(x=w938, y=w940) -> (x >= y?=w936:bool)
        n424 = local read "ct_Estufa"() -> (w926:dbl)
        n425 = case shown="True" w936 {
          tunnel: [FALSE w970] -> w930
          tunnel: w941 -> [w945 w952]
          tunnel: [w945 w963] -> w931
          tunnel: [w944 w962] -> w935
          tunnel: w934 -> [w944 _]
          tunnel: w926 -> [_ w956]
          tunnel: w925 -> [_ w954]
          tunnel: w924 -> [w943 w951]
          tunnel: w923 -> [w942 w950]
          tunnel: [w942 w949] -> w922
          tunnel: [w943 w948] -> w921
          frame False {
          }
          frame True {
            w960 = 1.0 ("y")
            # "um degC"
            # "Atualiza"
            # "Se já possui mais de duas leituras"
            # "Esta dentro da faixa desejada?"
            # "Entrou em regime permanente?"
            n426 = case shown="True" w954 {
              tunnel: [w983 w984] -> w953
              tunnel: w952 -> [w983 _]
              frame False {
              }
              frame True {
                n427 = flat-sequence {
                  tunnel: [w986] -> w985
                  tunnel: [w988] -> w984
                  tunnel: w985 -> [w988]
                  frame #0 {
                    n428 = local read "vecEstufa"() -> (w986:dbl[])
                  }
                  frame #1 {
                    n429 = local write "reset"(FALSE ("reset")) -> ()
                  }
                }
              }
            }
            n430 = local read "PV"() -> (w961:dbl)
            n431 = Build Array (concatenate)(w953, w961) -> (w969:dbl[])
            n432 = call "Is Value Changed.vim"("value"=w956) -> ("changed or first call?"=w955:bool)
            n433 = Array Subset(array=w969, index=1, length=3) -> (w963:dbl[])
            n434 = local write "increment"(w955) -> ()
            n435 = Array Max & Min(array=w963) -> (max value=w979:dbl, min value=w977:dbl)  [unwired: 2 out]
            n436 = local read "SP:"() -> (w959:dbl)
            n437 = Greater?(x=w956, y=2) -> (0:w964:bool)
            n438 = Subtract(x=w979, y=w977) -> (x-y=w978:dbl)
            n439 = Add(x=w959, y=w960) -> (x+y=w973:dbl)
            n440 = Subtract(x=w959, y=w960) -> (x-y=w974:dbl)
            n441 = local read "PV"() -> (w975:dbl)
            n442 = Greater Or Equal?(x=w975, y=w974) -> (x >= y?=w972:bool)
            n443 = Less Or Equal?(x=w975, y=w973) -> (x <= y?=w971:bool)
            n444 = Less Or Equal?(x=w978, y=w960) -> (x <= y?=w966:bool)
            n445 = And(x=w971, y=w972) -> (x .and. y?=w976:bool)
            n446 = And(x=w964, y=w966) -> (x .and. y?=w957:bool)
            n447 = local read "STOP"() -> (w958:bool)
            n448 = And(x=w957, y=w976) -> (x .and. y?=w947:bool)
            n449 = local write "STEADY?"(w957) -> ()
            n450 = disable-structure shown="Enabled" {
              disable-tunnel: [w981 w982] -> w970
              disable-tunnel: w958 -> [w980 w982]
              frame Disabled {
                n451 = Or(y=w980) -> (x .or. y?=w981:bool)  [unwired: 1 in]
              }
              frame Enabled {
              }
            }
            n452 = Send Notification(notification=w947, notifier=w950, error in (no error)=w951) -> (notifier out=w949:refnum<notifier>, error out=w948:errorcluster)
            n453 = Tick Count (ms)() -> (millisecond timer value=w962:u32)
          }
        }
        n454 = local read "STOP"() -> (w928:bool)
        n455 = Or(x=w930, y=w928) -> (x .or. y?=w929:bool)
      }
      n456 = disable-structure shown="Disabled" {
        disable-tunnel: w291 -> [w443 _]
        frame Disabled {
          n457 = while {
            tunnel: w443 -> [w445]
            stop <- w459 stop-if-true
            # "temp ambiente"
            # "temp estator 1"
            # "temp estator 2"
            # "tempo(s):"
            # "temp freio:"
            # "temp bobina1"
            # "temp bobina 2"
            # "Gerando log das temperaturas medidas no Dinamômetro"
            n458 = local read "temp pts"() -> (w446:T14)
            n459 = Unbundle(w446) -> ("t1 freio"=w452:dbl, "t2 bob 1"=w451:dbl, "t5 bob 2"=w450:dbl, "t4 estat 2"=w449:dbl, "t3 estat 1"=w448:dbl, "t6 amb"=w447:dbl)
            n460 = Wait (ms)(milliseconds to wait=u32 15000) -> ()  [unwired: 1 out]
            n461 = local read "t"() -> (w465:dbl)
            n462 = Number To Fractional String(number=w465, precision (6)=i16 3) -> (F-format string=w464:string)  [unwired: 2 in]
            n463 = Number To Fractional String(number=w452, precision (6)=i16 3) -> (F-format string=w463:string)  [unwired: 2 in]
            n464 = Number To Fractional String(number=w451, precision (6)=i16 3) -> (F-format string=w460:string)  [unwired: 2 in]
            n465 = Number To Exponential String(number=w450, precision (6)=i16 3) -> (E-format string=w468:string)  [unwired: 2 in]
            n466 = Number To Exponential String(number=w449, precision (6)=i16 3) -> (E-format string=w457:string)  [unwired: 2 in]
            n467 = Number To Exponential String(number=w448, precision (6)=i16 3) -> (E-format string=w454:string)  [unwired: 2 in]
            n468 = Number To Exponential String(number=w447, precision (6)=i16 3) -> (E-format string=w453:string)  [unwired: 2 in]
            n469 = Build Array(w464, w463, w460, w468, w457, w454, w453) -> (w461:string[])
            n470 = local read "STOP"() -> (w459:bool)
            n471 = call-poly <vilib>:"Write Delimited Spreadsheet.vi"("file path (dialog if empty)"=w445, "1D data"=w461, "append to file? (new file:F)"=TRUE, "transpose? (no:F)"=FALSE) -> ()  [unwired: 10 in, 2 out]
          }
        }
        frame Enabled {
        }
      }
      n472 = while {
        stop <- w904 stop-if-true
        # "Controle de Tabs - Escolha do Tipo de Ensaio Térmico"
        n473 = property on="Tab Control 9" class="TabCtl (strict)"() -> ("Pages"=w910:refnum<vi>[])  [unwired: 2 in, 2 out]
        n474 = local read "Tab Control 9"() -> (w905:enum32{"COMP_EVAL", "POWER MAP"})
        n475 = Index Array(array=w910, index #1=0 ("index"), index #2=1 ("index")) -> (element #1=w906:refnum<vi>, element #2=w907:refnum<vi>)
        n476 = case shown="\"COMP_EVAL\", Default" w905 {
          tunnel: w907 -> [w913 _]
          tunnel: w906 -> [_ w917]
          frame "COMP_EVAL", Default {
            # "Habilita aba atual e desabilita a outra"
            n477 = local read "Start EV?"() -> (w911:bool)
            n478 = Select(t=2.0, s=w911, f=0.0) -> (s? t:f=w912:dbl)
            n479 = property class="Page"(reference=w913, "PageEnb"=w912) -> ()  [unwired: 1 in, 2 out]
          }
          frame "POWER MAP" {
            n480 = local read "Start PMAP?"() -> (w916:bool)
            n481 = Select(t=2.0, s=w916, f=0.0) -> (s? t:f=w920:dbl)
            n482 = property class="Page"(reference=w917, "PageEnb"=w920) -> ()  [unwired: 1 in, 2 out]
          }
        }
        n483 = local read "STOP"() -> (w904:bool)
      }
      n484 = while {
        stop <- w993 stop-if-true
        # "Ensaio térmico automatizado"
        n485 = local read "Manual"() -> (w991:bool)
        n486 = local read "STOP"() -> (w992:bool)
        n487 = Or(x=w991, y=w992) -> (x .or. y?=w990:bool)
        n488 = Not(x=w990) -> (.not. x?=w989:bool)
        n489 = case shown="True" w989 {
          frame False {
            w994 = FALSE ("Automatic")
            # "nao habilita malha de controle externa"
            # "nao habilita malha de controle interna"
            # "Se manual estiver ligado"
            n490 = local write "CP EV ok"(w994) -> ()
            n491 = local write "PW MP ok"(w994) -> ()
          }
          frame True {
            # "Independentemente do tipo de ensaio, a condição da temperatura ambiente no interior da estufa deve ser respeitada!"
            # "Ligou motor, freio e ventilacao?\nEntao pode continuar o ensaio."
            n492 = local read "Continue"() -> (w995:bool)
            n493 = case shown="True" w995 {
              frame False {
              }
              frame True {
                # "Esta no modo Power Map"
                # "T_comp = SP?"
                # "TP MF ok"
                # "Ensaio de Comp. Eval?"
                n494 = local read "Start EV?"() -> (w996:bool)
                n495 = case shown="False" w996 {
                  frame False {
                  }
                  frame True {
                    # "Valor atual de velocidade"
                    # "Desabilita malha externa"
                    # "Liga controle da malha interna  gain scheduling"
                    n496 = local read "SP_Vel"() -> (w1005:i32)
                    n497 = local write "Velocidade (RPM)"(w1005) -> ()
                    n498 = local write "PW MP ok"(FALSE ("PW MP ok")) -> ()
                    n499 = local write "CP EV ok"(TRUE ("CP EV ok")) -> ()
                  }
                }
                n500 = local read "LIM SS MF"() -> (w1000:bool)
                n501 = local read "Start PMAP?"() -> (w999:bool)
                n502 = Not(x=w1000) -> (.not. x?=w997:bool)
                n503 = And(x=w997, y=w999) -> (x .and. y?=w998:bool)
                n504 = case shown="True" w998 {
                  tunnel: w996 -> [w1001 _]
                  frame False {
                    n505 = case shown="False" w1001 {
                      frame False {
                        # "componente atingiu o limite termico e o sistema\nestá no modo de ensaio Power Map?"
                        n506 = local write "PW MP ok"(FALSE ("PW MP ok")) -> ()
                      }
                      frame True {
                        # "nao esta no modo power map e \no modo comp eval esta ligado?\nnao faça nada"
                      }
                    }
                  }
                  frame True {
                    # "Desabilita malha interna"
                    # "Liga controle de temperatura (malha \nexterna)"
                    n507 = local write "CP EV ok"(FALSE ("CP EV ok")) -> ()
                    n508 = local write "PW MP ok"(TRUE ("PW MP ok")) -> ()
                  }
                }
              }
            }
          }
        }
        n509 = local read "STOP"() -> (w993:bool)
      }
      n510 = while {
        tunnel: [w699] -> w273
        tunnel: [w698] -> w272
        tunnel: [w697] -> w268
        tunnel: [w696] -> w267
        stop <- w700 stop-if-true
        # "Tratador de eventos manuais controlados pela IHM"
        n511 = event shown="[0] \"STOP\": Value Change" {
          selector: _ -> [_ _ _ _ _ _ _ _ _ _ _]
          dyn-events: _ -> [_ _ _ _ _ _ _ _ _ _ _]
          timeout: _ -> [_ _ _ _ _ _ _ _ _ _ _]
          tunnel: [w703 _ _ _ _ _ _ _ _ _ _] -> w700
          tunnel: [w702 _ _ _ _ _ _ _ _ _ _] -> w699
          tunnel: [w701 _ _ _ _ _ _ _ _ _ _] -> w698
          tunnel: [_ _ _ _ _ _ _ _ w805 _ _] -> w697
          tunnel: [_ _ _ _ _ _ _ _ w804 _ _] -> w696
          event "STOP": Value Change {
            n512 = event-data() -> ("NewVal"=w703:bool)  [unwired: 1 in, 5 out]
            n513 = flat-sequence {
              tunnel: [w746] -> w701
              tunnel: [w747] -> w702
              frame #0 {
                w704 = FALSE ("Automatic")
                # "Desabilita controle \nautomatico"
                n514 = local write "Start PMAP?"(w704) -> ()
                n515 = local write "PW MP ok"(w704) -> ()
                n516 = local write "CP EV ok"(w704) -> ()
                n517 = local write "Start EV?"(w704) -> ()
              }
              frame #1 {
                w705 = refnum<visa-resource-name> "Lambda" ("VISA name")
                # "mA --> A"
                # "Zera gradualmente a corrente\naplicada ao freio"
                n518 = local read "Corrente de saída"() -> (w706:dbl)
                n519 = while {
                  shift-right: [w709] -> _
                  shift-left: w706 -> [w710]
                  tunnel: w705 -> [w708]
                  tunnel: w705 -> [w707]
                  stop <- w711 stop-if-true
                  n520 = flat-sequence {
                    tunnel: w710 -> [w716]
                    tunnel: [w718] -> w709
                    tunnel: w708 -> [w715]
                    tunnel: w707 -> [w720]
                    frame #0 {
                      n521 = local write "Seta carga"(FALSE ("Status")) -> ()
                      n522 = Wait (ms)(milliseconds to wait=u32 2000) -> ()  [unwired: 1 out]
                    }
                    frame #1 {
                      n523 = Subtract(x=w716, y=0.05 ("x")) -> (x-y=w718:dbl)
                      n524 = call <instrlib>:"GENie Config Current Limit.vi"("Current Limit"=w718, "VISA"=w715) -> ()  [unwired: 8 in, 2 out]
                    }
                    frame #2 {
                      n525 = call <instrlib>:"GENie Meas Output Current.vi"("VISA"=w720) -> ("Output Current"=w719:dbl)  [unwired: 8 in, 2 out]
                      n526 = local write "Corrente de saída"(w719) -> ()
                      n527 = local write "Seta carga"(TRUE ("Seta carga")) -> ()
                      n528 = Wait (ms)(milliseconds to wait=u32 2000) -> ()  [unwired: 1 out]
                    }
                  }
                  n529 = Less Or Equal?(x=w709, y=0.0) -> (x <= y?=w711:bool)
                }
              }
              frame #2 {
                n530 = Wait (ms)(milliseconds to wait=u32 1500) -> ()  [unwired: 1 out]
              }
              frame #3 {
                # "para o motor"
                n531 = local read "Parâmetros serial"() -> (w727:T10)
                n532 = call "Serial_control.vi"("Enviar número"=u16 0, "Função"=T21."Set Speed", "comm cluster"=w727) -> ("translated message"=w726:string)  [unwired: 2 in, 3 out]
                n533 = local write "Tradução"(w726) -> ()
              }
              frame #4 {
                n534 = Wait (ms)(milliseconds to wait=u32 1000) -> ()  [unwired: 1 out]
              }
              frame #5 {
                w731 = refnum<k21> "resfriamento_freio"  # DAQmx Task Name
                w729 = FALSE ("Output ON")
                # "desliga freio, resfriamento do freio"
                n535 = local write "Liga Fonte"(w729) -> ()
                n536 = local write "Seta carga"(w729) -> ()
                n537 = call <instrlib>:"GENie Config Output On-Off.vi"("Output ON"=w729, "VISA"=refnum<visa-resource-name> "Lambda" ("VISA name")) -> ()  [unwired: 8 in, 2 out]
                n538 = call-poly <vilib>:"DAQmx Write.vi"("task/channels in"=w731, "data"=w729) -> ()  [unwired: 11 in, 3 out]
              }
              frame #6 {
                n539 = disable-structure shown="Disabled" {
                  frame Disabled {
                    # "Desliga a saída da fonte Extech"
                    n540 = flat-sequence {
                      tunnel: [w740] -> w736
                      tunnel: [w739] -> w735
                      tunnel: [w743] -> w734
                      tunnel: [w744] -> w733
                      tunnel: w736 -> [w744]
                      tunnel: w735 -> [w743]
                      frame #0 {
                        n541 = Wait (ms)(milliseconds to wait=u32 500) -> ()  [unwired: 1 out]
                      }
                      frame #1 {
                        n542 = local read "VISA name (EEC)"() -> (w741:refnum<visa-resource-name>)
                        n543 = local read "error in (EEC)"() -> (w738:errorcluster)
                        n544 = call "OFF (SubVI).vi"("error in (no error)"=w738, "VISA Refnum in"=w741) -> ("error out"=w739:errorcluster, "VISA Refnum out"=w740:refnum<visa-resource-name>)  [unwired: 8 in]
                      }
                      frame #2 {
                        n545 = Wait (ms)(milliseconds to wait=u32 500) -> ()  [unwired: 1 out]
                      }
                    }
                    n546 = VISA Close(VISA resource name=w733, error in (no error)=w734) -> (error out=w732:errorcluster)
                    n547 = local write "error Out (EEC)"(w732) -> ()
                  }
                  frame Enabled {
                  }
                }
              }
              frame #7 {
                n548 = Wait (ms)(milliseconds to wait=u32 250) -> ()  [unwired: 1 out]
              }
              frame #8 {
                # "desliga o ventilador"
                # "seta fonte 6812B para 0V"
                n549 = local read "VISA  name (6812B)"() -> (w753:refnum<visa-resource-name>)
                n550 = local read "error out (6812B)"() -> (w752:errorcluster)
                n551 = call <instrlib>:"Configure Voltage.vi"("VISA resource name"=w753, "Voltage Amplitude (1.0 V)"=0.0, "error in (no error)"=w752) -> ("VISA resource name out"=w750:refnum<visa-resource-name>, "error out"=w749:errorcluster)  [unwired: 11 in]
                n552 = call <instrlib>:"Enable Output.vi"("VISA resource name"=w750, "Enable Output (T: Enable)"=FALSE, "error in (no error)"=w749) -> ("VISA resource name out"=w747:refnum<visa-resource-name>, "error out"=w746:errorcluster)  [unwired: 11 in]
              }
            }
          }
          event "Gains_L1.integral time (Ti, min)": Value Change {
            n553 = event-data() -> ("NewVal"=w754:dbl)  [unwired: 1 in, 5 out]
            n554 = disable-structure shown="Disabled" {
              disable-tunnel: w754 -> [w757 _]
              frame Disabled {
                # "Atualiza ganho Ti do controlador do componente L100"
                n555 = Multiply(x=w757, y=60.0) -> (x*y=w755:dbl)
                n556 = local write "zF_L1_i"(w755) -> ()
                n557 = local write "zF_L1"(w755) -> ()
              }
              frame Enabled {
              }
            }
          }
          event "Gains_C5.integral time (Ti, min)": Value Change {
            n558 = event-data() -> ("NewVal"=w758:dbl)  [unwired: 1 in, 5 out]
            n559 = disable-structure shown="Disabled" {
              disable-tunnel: w758 -> [w761 _]
              frame Disabled {
                # "Atualiza ganho Ti do controlador do componenteC504"
                n560 = Multiply(x=w761, y=60.0) -> (x*y=w759:dbl)
                n561 = local write "zF_C5_i"(w759) -> ()
                n562 = local write "zF_C5"(w759) -> ()
              }
              frame Enabled {
              }
            }
          }
          event "Gains_C1.integral time (Ti, min)": Value Change {
            n563 = event-data() -> ("NewVal"=w762:dbl)  [unwired: 1 in, 5 out]
            n564 = disable-structure shown="Disabled" {
              disable-tunnel: w762 -> [w765 _]
              frame Disabled {
                # "Atualiza ganho Ti do controlador do componente C011"
                n565 = Multiply(x=w765, y=60.0) -> (x*y=w763:dbl)
                n566 = local write "zF_C1_i"(w763) -> ()
                n567 = local write "zF_C1"(w763) -> ()
              }
              frame Enabled {
              }
            }
          }
          event "Gains_MIC.integral time (Ti, min)": Value Change {
            n568 = event-data() -> ("NewVal"=w766:dbl)  [unwired: 1 in, 5 out]
            n569 = disable-structure shown="Disabled" {
              disable-tunnel: w766 -> [w769 _]
              frame Disabled {
                # "Atualiza ganho Ti do controlador do componente MIC601"
                n570 = Multiply(x=w769, y=60.0) -> (x*y=w767:dbl)
                n571 = local write "zF_MIC_i"(w767) -> ()
                n572 = local write "zF_MIC"(w767) -> ()
              }
              frame Enabled {
              }
            }
          }
          event "Parar motor": Value Change {
            # "Por segurança, pode fazer quando quiser"
            n573 = event-data() -> ()  [unwired: 1 in, 6 out]
            n574 = flat-sequence {
              frame #0 {
                w770 = FALSE ("Loop 2 Access?")
                n575 = local write "Enviar velocidade"(w770) -> ()
                n576 = local write "Envia mensagem"(w770) -> ()
              }
              frame #1 {
                # "Envia referência de velocidade zero (0 RPM) para o motor"
                n577 = local read "Parâmetros serial"() -> (w775:T10)
                n578 = local write "Velocidade (RPM)"(u16 0 ("Velocidade (RPM)")) -> ()
                n579 = call "Serial_control.vi"("Enviar número"=u16 0, "Função"=T21."Set Speed", "comm cluster"=w775) -> ("translated message"=w776:string)  [unwired: 2 in, 3 out]
                n580 = local write "Tradução"(w776) -> ()
                n581 = Wait (ms)(milliseconds to wait=u32 1000) -> ()  [unwired: 1 out]
              }
            }
          }
          event "Enviar velocidade": Value Change {
            n582 = event-data() -> ()  [unwired: 1 in, 6 out]
            n583 = local read "Manual"() -> (w777:bool)
            n584 = case shown="True" w777 {
              frame False {
                n585 = local read "Parâmetros serial"() -> (w780:T10)
                n586 = call "Serial_control.vi"("Enviar número"=u16 0, "Função"=T21."Set Speed", "comm cluster"=w780) -> ("translated message"=w781:string)  [unwired: 2 in, 3 out]
                n587 = local write "Tradução"(w781) -> ()
              }
              frame True {
                n588 = flat-sequence {
                  frame #0 {
                    w782 = FALSE ("Loop 2 Access?")
                    n589 = local write "Parar motor"(w782) -> ()
                    n590 = local write "Envia mensagem"(w782) -> ()
                  }
                  frame #1 {
                    # "Envia a referência de velocidade (em RPM) para o inversor"
                    n591 = local read "Velocidade (RPM)"() -> (w783:u16)
                    n592 = local read "Parâmetros serial"() -> (w785:T10)
                    n593 = call "Serial_control.vi"("Enviar número"=w783, "Função"=T21."Set Speed", "comm cluster"=w785) -> ("translated message"=w786:string)  [unwired: 2 in, 3 out]
                    n594 = local write "Tradução"(w786) -> ()
                  }
                  frame #2 {
                    n595 = while {
                      stop <- w787 stop-if-true
                      n596 = local read "Velocidade (RPM)"() -> (w791:u16)
                      n597 = local read "Vel Real"() -> (w792:u16)
                      n598 = Greater Or Equal?(x=w792, y=w791) -> (x >= y?=w790:bool)
                      n599 = case shown="True" w790 {
                        selector: w790 -> [_ w794]
                        tunnel: [FALSE w794] -> w789
                        frame False {
                        }
                        frame True {
                        }
                      }
                      n600 = local read "STOP"() -> (w788:bool)
                      n601 = Or(x=w789, y=w788) -> (x .or. y?=w787:bool)
                    }
                  }
                  frame #3 {
                    n602 = local write "Enviar velocidade"(FALSE ("Enviar velocidade")) -> ()
                  }
                }
              }
            }
          }
          event "Envia mensagem": Value Change {
            n603 = event-data() -> ()  [unwired: 1 in, 6 out]
            n604 = flat-sequence {
              frame #0 {
                w796 = FALSE ("Loop 2 Access?")
                n605 = local write "Parar motor"(w796) -> ()
                n606 = local write "Enviar velocidade"(w796) -> ()
              }
              frame #1 {
                # "Envia mensagem (em hexadecimal) para o inversor"
                n607 = local read "Parâmetros serial"() -> (w800:T10)
                n608 = call "Serial_control.vi"("Message"="Mensagem", "Função"=T21."Send Static Message", "comm cluster"=w800) -> ("translated message"=w801:string)  [unwired: 2 in, 3 out]
                n609 = local write "Tradução"(w801) -> ()
                n610 = Wait (ms)(milliseconds to wait=u32 500) -> ()  [unwired: 1 out]
              }
            }
          }
          event "Voltage Amplitude (1.0 V)": Value Change {
            n611 = event-data() -> ("NewVal"=w803:dbl)  [unwired: 1 in, 5 out]
            n612 = local read "Muda tensao"() -> (w802:bool)
            n613 = case shown="True" w802 {
              tunnel: [w807 w810] -> w805
              tunnel: [errorcluster {"status"=FALSE, "code"=0, "source"=""} ("error out") w809] -> w804
              tunnel: w803 -> [_ w808]
              frame False {
                n614 = local read "VISA  name (6812B)"() -> (w807:refnum<visa-resource-name>)
              }
              frame True {
                w830 = 1 items=["Immediate", "Bus", "External", "Phase", "Trigger Out"]  # Trigger Source
                w829 = 1 items=["Output"=1, "Synchronous Source"=2, "Measurement"=3]  # Trigger Sequence
                # "cfg Voltage -> cfg Trigger -> cfg Pulse -> Enable Output -> Meas P&C"
                # "Se o operador quiser mudar a tensao da fonte  6812B manualmente"
                n615 = local read "Triggered Voltage Amplitude (V)"() -> (w814:dbl)
                n616 = local read "VISA  name (6812B)"() -> (w828:refnum<visa-resource-name>)
                n617 = local read "error out (6812B)"() -> (w827:errorcluster)
                n618 = call <instrlib>:"Configure Voltage.vi"("VISA resource name"=w828, "Triggered Voltage Amplitude (1.0 V)"=w814, "Voltage Amplitude (1.0 V)"=w808, "error in (no error)"=w827) -> ("VISA resource name out"=w822:refnum<visa-resource-name>, "error out"=w821:errorcluster)  [unwired: 10 in]
                n619 = call <instrlib>:"Configure Trigger.vi"("VISA resource name"=w822, "Trigger Sequence (1: Output 1)"=w830, "Trigger Source (0: Immediate)"=w829, "error in (no error)"=w821, "Trigger Delay (0 s)"="Trigger Delay (s)") -> ("VISA resource name out"=w823:refnum<visa-resource-name>, "error out"=w824:errorcluster)  [unwired: 9 in]
                n620 = call <instrlib>:"Configure Pulse.vi"("VISA resource name"=w823, "Pulse Count (1)"="Pulse Count", "Period (0.0333 s)"="Period (s)", "error in (no error)"=w824, "Pulse Characteristic (0: Duty Cycle)"="Pulse Characteristic", "Pulse Characteristic Value (50)"="Pulse Characteristic Value (%)") -> ("VISA resource name out"=w820:refnum<visa-resource-name>, "error out"=w819:errorcluster)  [unwired: 8 in]
                n621 = call <instrlib>:"Enable Output.vi"("VISA resource name"=w820, "error in (no error)"=w819) -> ("VISA resource name out"=w826:refnum<visa-resource-name>, "error out"=w825:errorcluster)  [unwired: 12 in]
                n622 = call "measPwrCur.vi"("VISA resource name"=w826, "error in (no error)"=w825) -> ("VolMeas"=→"VolMeas":cluster{"AC + DC RMS Voltage":dbl}, "CurMeas"=→"CurMeas":T24, "VISA resource name out"=w810:refnum<visa-resource-name>, "PwrMeas"=→"PwrMeas":cluster{"Total Power":dbl, "Power Factor":dbl}, "error out"=w809:errorcluster)  [unwired: 2 in]
              }
            }
          }
          event "Seta carga": Value Change {
            # "Corrente aplicada ao freio é o valor setado pelo operador (manual) ou calculado pelo sistema de controle"
            n623 = event-data() -> ()  [unwired: 1 in, 6 out]
            n624 = local read "Manual"() -> (w833:bool)
            n625 = case shown="True" w833 {
              tunnel: [0.0 ("Limite de corrente") w839] -> w834
              frame False {
              }
              frame True {
                n626 = local read "Limite de corrente"() -> (w839:dbl)
              }
            }
            n627 = call <instrlib>:"GENie Config Current Limit.vi"("Current Limit"=w834, "VISA"=refnum<visa-resource-name> "Lambda" ("VISA name")) -> ("VISA out"=w836:refnum<visa-resource-name>)  [unwired: 8 in, 1 out]
            n628 = local read "Limite de tensão"() -> (w837:dbl)
            n629 = call <instrlib>:"GENie Config Voltage Limit.vi"("Volt Limit"=w837, "VISA"=w836) -> ()  [unwired: 8 in, 2 out]
            n630 = local write "Seta carga"(FALSE ("Seta carga")) -> ()
          }
          event "Liga Fonte": Value Change {
            w842 = refnum<k21> "resfriamento_freio"  # DAQmx Task Name
            # "Liga fonte de corrente e o sistema pneumático para resfriamento do freio"
            n631 = event-data() -> ("NewVal"=w841:bool)  [unwired: 1 in, 5 out]
            n632 = call <instrlib>:"GENie Config Output On-Off.vi"("Output ON"=w841, "VISA"=refnum<visa-resource-name> "Lambda" ("VISA name")) -> ()  [unwired: 8 in, 2 out]
            n633 = call-poly <vilib>:"DAQmx Write.vi"("task/channels in"=w842, "data"=w841) -> ()  [unwired: 11 in, 3 out]
          }
        }
      }
      n634 = while {
        stop <- w649 stop-if-true
        # "Se a estufa está com a temperatura ambiente, executa rotina de inicialização do controle automatico"
        n635 = local read "Continue"() -> (w646:bool)
        n636 = local read "LIM SS"() -> (w648:bool)
        n637 = Not(x=w646) -> (.not. x?=w645:bool)
        n638 = And(x=w648, y=w645) -> (x .and. y?=w647:bool)
        n639 = case shown="True" w647 {
          frame False {
          }
          frame True {
            # "Qual modo de ensaio?"
            n640 = local read "Start PMAP?"() -> (w650:bool)
            n641 = local read "Start EV?"() -> (w652:bool)
            n642 = Or(x=w652, y=w650) -> (x .or. y?=w651:bool)
            n643 = case shown="True" w651 {
              tunnel: w652 -> [_ w655]
              frame False {
                # "Se nenhum dos dois modos foi acionado, entao deixa motor desligado e nao continua nenhum dos dois ensaios no modo automatico"
                n644 = disable-structure shown="Disabled" {
                  frame Disabled {
                    n645 = local write "Velocidade (RPM)"(u16 0 ("Velocidade (RPM)")) -> ()
                  }
                  frame Enabled {
                  }
                }
                n646 = local write "Continue"(FALSE ("Continue")) -> ()
              }
              frame True {
                n647 = flat-sequence {
                  tunnel: w655 -> [w656]
                  frame #0 {
                    # "desabilita botao"
                    # "Liga o motor com a velocidade desejada para o ensaio atual"
                    n648 = case shown="False" w656 {
                      tunnel: [u16 3500 ("Velocidade (RPM)") w660] -> w657
                      frame False {
                        # "Modo Pwr Map"
                      }
                      frame True {
                        # "SP da primeira condicao\ndo teste"
                        # "Modo COMP EVAL"
                        n649 = local read "SP_Vel"() -> (w660:i32)
                      }
                    }
                    n650 = local write "Velocidade (RPM)"(w657) -> ()
                    n651 = local write "Parar motor"(FALSE ("Parar motor")) -> ()
                  }
                  frame #1 {
                    # "Espera motor partir e a velocidade assentar"
                    n652 = local read "Parâmetros serial"() -> (w662:T10)
                    n653 = local read "Velocidade (RPM)"() -> (w661:u16)
                    n654 = call "Serial_control.vi"("Enviar número"=w661, "Função"=T21."Set Speed", "comm cluster"=w662) -> ("translated message"=w664:string)  [unwired: 2 in, 3 out]
                    n655 = local write "Tradução"(w664) -> ()
                  }
                  frame #2 {
                    # "Verifica se motor atingiu a velocidade desejada:"
                    n656 = while {
                      stop <- w666 stop-if-true
                      n657 = local read "Velocidade (RPM)"() -> (w669:u16)
                      n658 = local read "Vel Real"() -> (w670:u16)
                      n659 = Greater Or Equal?(x=w670, y=w669) -> (x >= y?=w668:bool)
                      n660 = case shown="True" w668 {
                        selector: w668 -> [_ w672]
                        tunnel: [FALSE w672] -> w667
                        frame False {
                        }
                        frame True {
                        }
                      }
                      n661 = local read "STOP"() -> (w665:bool)
                      n662 = Or(x=w667, y=w665) -> (x .or. y?=w666:bool)
                    }
                  }
                  frame #3 {
                    w674 = refnum<k21> "resfriamento_freio"  # DAQmx Task Name
                    # "Liga o resfriamento do freio"
                    n663 = call-poly <vilib>:"DAQmx Write.vi"("task/channels in"=w674, "data"=TRUE) -> ()  [unwired: 11 in, 3 out]
                  }
                  frame #4 {
                    w675 = u32 500  # Interval
                    n664 = Wait (ms)(milliseconds to wait=w675) -> ()  [unwired: 1 out]
                  }
                  frame #5 {
                    n665 = disable-structure shown="Disabled" {
                      frame Disabled {
                        # "Liga ventilação do motor"
                        n666 = local read "VISA  name (6812B)"() -> (w681:refnum<visa-resource-name>)
                        n667 = local read "error out (6812B)"() -> (w680:errorcluster)
                        n668 = call <instrlib>:"Configure Voltage.vi"("VISA resource name"=w681, "Voltage Amplitude (1.0 V)"=220.0, "error in (no error)"=w680) -> ("VISA resource name out"=w679:refnum<visa-resource-name>, "error out"=w678:errorcluster)  [unwired: 11 in]
                        n669 = call <instrlib>:"Enable Output.vi"("VISA resource name"=w679, "Enable Output (T: Enable)"=TRUE, "error in (no error)"=w678) -> ()  [unwired: 11 in, 2 out]
                      }
                      frame Enabled {
                      }
                    }
                  }
                  frame #6 {
                    # "Continuar ensaio"
                    n670 = local write "Continue"(TRUE ("Continue")) -> ()
                  }
                }
              }
            }
          }
        }
        n671 = local read "STOP"() -> (w649:bool)
      }
      n672 = while {
        stop <- w683 stop-if-true
        n673 = local read "LIM SS"() -> (w686:bool)
        n674 = local read "STEADY?"() -> (w685:bool)
        n675 = local read "STOP"() -> (w683:bool)
        n676 = Not(x=w686) -> (.not. x?=w684:bool)
        n677 = And(x=w685, y=w684) -> (x .and. y?=w687:bool)
        n678 = case shown="True" w687 {
          frame False {
          }
          frame True {
            n679 = disable-structure shown="Disabled" {
              frame Disabled {
                n680 = local write "ct_Estufa"(0.0 ("counter")) -> ()
              }
              frame Enabled {
              }
            }
            n681 = local write "vecEstufa"(dbl[] [-999.0, -999.0, -999.0] ("Vetor Leituras")) -> ()
            n682 = local write "reset"(TRUE ("reset")) -> ()
          }
        }
      }
      n683 = while {
        tunnel: [w1351] -> w304
        tunnel: [w1296] -> w303
        tunnel: w302 -> [w1290]
        i -> [w1295]
        stop <- w1354 stop-if-true
        # "era 1000"
        # "limpa erro"
        # "limpa erro"
        # "temp. do termopar a ser controlada pelo controlador Ens. Ter. em MF"
        # "PT100"
        # "DAQ Temperatura Termopares do  IF e dos PT100 de Temperatura  do Forno e do Dinamômetro"
        n684 = call <vilib>:"High Resolution Polling Wait.vi"("seconds to wait"=1.0) -> ()  [unwired: 10 in, 1 out]
        n685 = call <instrlib>:"EZ Temperature.vi"("VISA Resource Name"=w1290, "Scan List (empty)"="301,302,303,305,306,307,308,310,311,312,313,315", "Transducer Type (4:Def-Last)"=T23."Thermocouple") -> ("VISA Resource Name Out"=w1351:refnum<visa-resource-name>, "Output Array"=w1357:dbl[], "error out"=w1289:errorcluster)  [unwired: 10 in]
        n686 = Unbundle By Name(w1289) -> ("code"=w1284:i32)
        n687 = call <vilib>:"Clear Errors.vi"("error in (no error)"=w1289, "specific error code to clear (0: all)"=w1284) -> ("error out"=→"error out TC":errorcluster)  [unwired: 4 in, 1 out]
        n688 = Index Array(array=w1357, index #1=0 ("index"), index #2=1 ("index"), index #3=2 ("index"), index #4=3 ("index"), index #5=4 ("index"), index #6=5 ("index"), index #7=6 ("index"), index #8=7 ("index"), index #9=8 ("index"), index #10=9 ("index"), index #11=10 ("index"), index #12=11 ("index")) -> (element #1=w1293:dbl, element #3=w1328:dbl, element #4=w1294:dbl, element #5=w1327:dbl, element #6=w1326:dbl, element #7=w1325:dbl, element #8=w1324:dbl, element #9=w1323:dbl, element #10=w1322:dbl, element #11=w1280:dbl, element #12=w1321:dbl)  [unwired: 1 out]
        n689 = local write "TP 1"(w1293) -> ()
        n690 = local write "TP 3"(w1328) -> ()
        n691 = local write "TP 5"(w1294) -> ()
        n692 = local write "TP 6"(w1327) -> ()
        n693 = local write "TP 7"(w1326) -> ()
        n694 = local write "TP 8"(w1325) -> ()
        n695 = local write "TP 10"(w1324) -> ()
        n696 = local write "TP 11"(w1323) -> ()
        n697 = local write "TP 12"(w1322) -> ()
        n698 = local write "TP 13"(w1280) -> ()
        n699 = local write "TP 15"(w1321) -> ()
        n700 = Bundle(w1293, "index"=95) -> (→"G. TP 1":cluster{dbl, "index":i32})  [unwired: 1 in]
        n701 = Bundle(w1294, "index"=95) -> (→"G. TP 5":cluster{dbl, "index":i32})  [unwired: 1 in]
        n702 = Bundle(w1323, "index"=95) -> (→"G. TP 11":cluster{dbl, "index":i32})  [unwired: 1 in]
        n703 = Bundle(w1322, "index"=95) -> (→"G. TP 12":cluster{dbl, "index":i32})  [unwired: 1 in]
        n704 = Bundle(w1280, "index"=95) -> (→"G. TP 13":cluster{dbl, "index":i32})  [unwired: 1 in]
        n705 = Bundle(w1321, "index"=80) -> (→"G. TP 15":cluster{dbl, "index":i32})  [unwired: 1 in]
        n706 = Bundle(w1328, "index"=110) -> (→"G. TP 3":cluster{dbl, "index":i32})  [unwired: 1 in]
        n707 = Bundle(w1327, "index"=115) -> (→"G. TP 6":cluster{dbl, "index":i32})  [unwired: 1 in]
        n708 = Bundle(w1326, "index"=115) -> (→"G. TP 7":cluster{dbl, "index":i32})  [unwired: 1 in]
        n709 = Bundle(w1325, "index"=115) -> (→"G. TP 8":cluster{dbl, "index":i32})  [unwired: 1 in]
        n710 = Bundle(w1324, "index"=100) -> (→"G. TP 10":cluster{dbl, "index":i32})  [unwired: 1 in]
        n711 = local write "PV_MIC"(w1280) -> ()
        n712 = call-poly <vilib>:"Random Number (Range).vi"("lower bound (0)"=0.01, "upper bound (100)"=0.21) -> ("number"=w1285:dbl)  [unwired: 9 in]
        n713 = Add(x=w1293, y=w1285) -> (x+y=w1292:dbl)
        n714 = local write "TP 2"(w1292) -> ()
        n715 = call <instrlib>:"EZ Temperature.vi"("VISA Resource Name"=w1290, "Scan List (empty)"="101,102,103, 104, 105, 106, 304,309", "Transducer Type (4:Def-Last)"=T23."4-Wire RTD") -> ("VISA Resource Name Out"=w1296:refnum<visa-resource-name>, "Output Array"=w1308:dbl[], "error out"=w1288:errorcluster)  [unwired: 10 in]
        n716 = Index Array(array=w1308, index #1=0 ("index"), index #2=1 ("index"), index #3=2 ("index"), index #4=3 ("index"), index #5=4 ("index"), index #6=5 ("index"), index #7=6 ("index"), index #8=7 ("index")) -> (element #1=w1312:dbl, element #2=w1313:dbl, element #3=w1314:dbl, element #4=w1315:dbl, element #5=w1316:dbl, element #6=w1317:dbl, element #7=w1318:dbl, element #8=w1319:dbl)
        n717 = Bundle(w1292, "index"=95) -> (→"G. TP 2":cluster{dbl, "index":i32})  [unwired: 1 in]
        n718 = Unbundle By Name(w1288) -> ("code"=w1282:i32)
        n719 = disable-structure shown="Disabled" {
          disable-tunnel: w1317 -> [w1375 _]
          disable-tunnel: w1316 -> [w1374 _]
          disable-tunnel: w1315 -> [w1373 _]
          disable-tunnel: w1314 -> [w1372 _]
          disable-tunnel: w1313 -> [w1371 _]
          disable-tunnel: w1312 -> [w1370 _]
          frame Disabled {
            n720 = Bundle(w1370, w1371, w1372, w1373, w1374, w1375) -> (→"Chart Temperatura":cluster{dbl, dbl, dbl, dbl, dbl, dbl})  [unwired: 1 in]
          }
          frame Enabled {
          }
        }
        n721 = local write "PT100_CH4"(w1318) -> ()
        n722 = local write "PT100_CH9"(w1319) -> ()
        n723 = Add(x=w1318, y=w1319) -> (x+y=w1309:dbl)
        n724 = Bundle(w1312, w1313, w1314, w1315, w1316, w1317) -> (→"temp pts":cluster{dbl, dbl, dbl, dbl, dbl, dbl})  [unwired: 1 in]
        n725 = call <vilib>:"Clear Errors.vi"("error in (no error)"=w1288, "specific error code to clear (0: all)"=w1282) -> ("error out"=→"error out Pt100":errorcluster)  [unwired: 4 in, 1 out]
        n726 = local read "STOP"() -> (w1354:bool)
        n727 = Divide(x=w1309, y=2.0) -> (x/y=w1310:dbl)
        n728 = Wait (ms)(milliseconds to wait=u32 1000 ("millisecond multiple")) -> ()  [unwired: 1 out]
        n729 = local write "PV"(w1310) -> ()
        "Iteration" <- w1295
      }
      n730 = call <vilib>:"High Resolution Relative Seconds.vi"() -> ("relative seconds"=w259:dbl)
      n731 = while {
        tunnel: w259 -> [w475]
        stop <- w473 stop-if-true
        n732 = call <vilib>:"High Resolution Relative Seconds.vi"() -> ("relative seconds"=w476:dbl)
        n733 = Subtract(x=w476, y=w475) -> (x-y=w474:dbl)
        n734 = local write "Time"(w474) -> ()
        n735 = local read "STOP"() -> (w473:bool)
        n736 = Wait (ms)(milliseconds to wait=u32 10) -> ()  [unwired: 1 out]
      }
      n737 = while {
        tunnel: refnum<visa-resource-name> "Lambda" ("VISA name") -> [w1223]
        stop <- w1222 stop-if-true
        # "era 200"
        # "Aquisição - Fonte DC Lambda"
        n738 = call <instrlib>:"GENie Meas Output Voltage.vi"("VISA"=w1223) -> ("Output Voltage"=→"Tensão de saída":dbl, "VISA out"=w1226:refnum<visa-resource-name>)  [unwired: 8 in, 1 out]
        n739 = call <instrlib>:"GENie Meas Output Current.vi"("VISA"=w1226) -> ("Output Current"=→"Corrente de saída":dbl)  [unwired: 8 in, 2 out]
        n740 = local read "STOP"() -> (w1222:bool)
        n741 = Wait (ms)(milliseconds to wait=u32 1000) -> ()  [unwired: 1 out]
      }
      n742 = while {
        stop <- w1505 stop-if-true
        # "Malha de controle de Temperatura da Estufa  - PI"
        n743 = local read "PV"() -> (w1509:dbl)
        n744 = Bundle("PV"=w1509, "SP:"="SP:") -> (→"Process variable and Setpoint":cluster{"PV":dbl, "SP:":dbl})  [unwired: 1 in]
        n745 = call-poly <vilib>:"PID.vi"("output range"=cluster{"output high":dbl, "output low":dbl} {"output high"=99.9, "output low"=0.01}, "PID gains"="PID gains", "process variable"=w1509, "setpoint"="SP:") -> ("output"=w1504:dbl)  [unwired: 6 in, 1 out]
        n746 = local write "Duty Cycle"(w1504) -> ()
        n747 = Multiply(x="Ts", y=u32 1000 ("unsigned 32bit integer")) -> (x*y=w1503:dbl)
        n748 = local read "STOP"() -> (w1505:bool)
        n749 = Wait Until Next ms Multiple(millisecond multiple=w1503) -> ()  [unwired: 1 out]
        n750 = disable-structure shown="Disabled" {
          disable-tunnel: w1504 -> [w1513 _]
          frame Disabled {
            "MV" <- w1513
          }
          frame Enabled {
          }
        }
      }
      n751 = while {
        shift-right: [w846] -> _
        shift-left: 0.0 -> [w845]
        stop <- w843 stop-if-true
        # "Contador de leituras do vector de temps da estufa"
        n752 = local read "increment"() -> (w844:bool)
        n753 = case shown="True" w844 {
          tunnel: [w847 w849] -> w846
          tunnel: w845 -> [w847 w848]
          frame False {
          }
          frame True {
            n754 = flat-sequence {
              tunnel: w848 -> [w851]
              tunnel: [w850] -> w849
              frame #0 {
                n755 = Increment(x=w851) -> (x+1=w850:dbl)
                n756 = local write "ct_Estufa"(w850) -> ()
              }
              frame #1 {
                n757 = local write "increment"(FALSE ("increment")) -> ()
              }
            }
          }
        }
        n758 = local read "STOP"() -> (w843:bool)
      }
      n759 = Release Notifier(notifier=w276, error in (no error)=w275) -> ()  [unwired: 1 in, 3 out]
      n760 = local read "vecTempME"() -> (w253:dbl[])
      n761 = Obtain Notifier(notification data type=FALSE) -> (notifier out=w250:refnum<notifier>, error out=w251:errorcluster)  [unwired: 3 in, 1 out]
      n762 = call <instrlib>:"Close.vi"("VISA Resource Name"=w303) -> ()  [unwired: 14 in, 1 out]
      n763 = call <instrlib>:"Close.vi"("VISA Resource Name"=w304) -> ()  [unwired: 14 in, 1 out]
      n764 = while {
        shift-right: [w391] -> _
        shift-left: w253 -> [w401]
        shift-right: [w395] -> _
        shift-left: _ -> [w394]
        tunnel: w251 -> [w387]
        tunnel: w250 -> [w386]
        tunnel: [w385] -> w248
        tunnel: [w384] -> w247
        stop <- w383 stop-if-true
        # "ms"
        # "ms"
        # "s"
        # "Verifica se a temperatura da estufa atingiu o regime permanente"
        n765 = local read "TBRMF(min)"() -> (w390:u32)
        n766 = Tick Count (ms)() -> (millisecond timer value=w397:u32)
        n767 = local read "Res_TempME"() -> (w388:bool)
        n768 = Multiply(x=w390, y=u32 60) -> (x*y=w392:u32)
        n769 = Subtract(x=w397, y=w394) -> (x-y=w398:u32)
        n770 = Multiply(x=w392, y=u32 1000) -> (x*y=w400:u32)
        n771 = Greater Or Equal?(x=w398, y=w400) -> (x >= y?=w396:bool)
        n772 = local read "ct_TempME"() -> (w389:dbl)
        n773 = case shown="True" w396 {
          tunnel: w401 -> [w405 w411]
          tunnel: [w405 w421] -> w391
          tunnel: [w404 w420] -> w395
          tunnel: w394 -> [w404 _]
          tunnel: w389 -> [_ w415]
          tunnel: w388 -> [_ w413]
          tunnel: w387 -> [w403 w406]
          tunnel: w386 -> [w402 w410]
          tunnel: [w402 w409] -> w385
          tunnel: [w403 w408] -> w384
          frame False {
            (unwired) FALSE
          }
          frame True {
            w418 = 0.5 ("y")
            # "meio degC"
            # "Atualiza"
            # "Se já possui mais de duas leituras"
            # "Esta dentro da faixa desejada?"
            # "Entrou em regime permanente?"
            n774 = case shown="True" w413 {
              tunnel: [w437 w438] -> w412
              tunnel: w411 -> [w437 _]
              frame False {
              }
              frame True {
                n775 = flat-sequence {
                  tunnel: [w440] -> w439
                  tunnel: [w442] -> w438
                  tunnel: w439 -> [w442]
                  frame #0 {
                    n776 = local read "vecTempME"() -> (w440:dbl[])
                  }
                  frame #1 {
                    n777 = local write "Res_TempME"(FALSE ("reset")) -> ()
                  }
                }
              }
            }
            n778 = local read "PV_MIC"() -> (w419:dbl)
            n779 = Build Array (concatenate)(w412, w419) -> (w427:dbl[])
            n780 = call "Is Value Changed.vim"("value"=w415) -> ("changed or first call?"=w414:bool)
            n781 = local write "INC_TempME"(w414) -> ()
            n782 = Array Subset(array=w427, index=1, length=3) -> (w421:dbl[])
            n783 = Array Max & Min(array=w421) -> (max value=w436:dbl, min value=w434:dbl)  [unwired: 2 out]
            n784 = local read "SP_MIC"() -> (w417:dbl)
            n785 = Greater?(x=w415, y=2) -> (0:w422:bool)
            n786 = Subtract(x=w436, y=w434) -> (x-y=w435:dbl)
            n787 = Add(x=w417, y=w418) -> (x+y=w430:dbl)
            n788 = Subtract(x=w417, y=w418) -> (x-y=w431:dbl)
            n789 = local read "PV_MIC"() -> (w432:dbl)
            n790 = Greater Or Equal?(x=w432, y=w431) -> (x >= y?=w429:bool)
            n791 = Less Or Equal?(x=w432, y=w430) -> (x <= y?=w428:bool)
            n792 = Less Or Equal?(x=w435, y=w418) -> (x <= y?=w424:bool)
            n793 = And(x=w428, y=w429) -> (x .and. y?=w433:bool)
            n794 = And(x=w422, y=w424) -> (x .and. y?=w416:bool)
            n795 = And(x=w416, y=w433) -> (x .and. y?=w407:bool)
            n796 = local write "STEADY MF?"(w416) -> ()
            n797 = Send Notification(notification=w407, notifier=w410, error in (no error)=w406) -> (notifier out=w409:refnum<notifier>, error out=w408:errorcluster)
            n798 = Tick Count (ms)() -> (millisecond timer value=w420:u32)
          }
        }
        n799 = local read "STOP"() -> (w383:bool)
      }
      n800 = while {
        tunnel: w250 -> [w378]
        stop <- w380 stop-if-true
        n801 = Wait on Notification(notifier=w378) -> (notification=w379:bool, error out=w380:errorcluster)  [unwired: 3 in, 2 out]
        n802 = case shown="False" w379 {
          frame False {
            n803 = local write "LIM SS MF"(FALSE ("Boolean 2")) -> ()
          }
          frame True {
            n804 = local write "LIM SS MF"(TRUE ("Boolean 2")) -> ()
          }
        }
      }
      n805 = while {
        shift-right: [w485] -> _
        shift-left: 0.0 -> [w484]
        stop <- w482 stop-if-true
        # "Contador de leituras"
        n806 = local read "INC_CEVAL"() -> (w483:bool)
        n807 = case shown="True" w483 {
          tunnel: [w486 w488] -> w485
          tunnel: w484 -> [w486 w487]
          frame False {
          }
          frame True {
            n808 = flat-sequence {
              tunnel: w487 -> [w490]
              tunnel: [w489] -> w488
              frame #0 {
                n809 = Increment(x=w490) -> (x+1=w489:dbl)
                n810 = local write "ct_CEVAL"(w489) -> ()
              }
              frame #1 {
                n811 = local write "INC_CEVAL"(FALSE ("increment")) -> ()
              }
            }
          }
        }
        n812 = local read "STOP"() -> (w482:bool)
      }
      n813 = Obtain Notifier(notification data type=FALSE) -> (notifier out=w260:refnum<notifier>, error out=w263:errorcluster)  [unwired: 3 in, 1 out]
      n814 = while {
        tunnel: w260 -> [w477]
        stop <- w479 stop-if-true
        n815 = Wait on Notification(notifier=w477) -> (notification=w478:bool, error out=w479:errorcluster)  [unwired: 3 in, 2 out]
        n816 = case shown="True" w478 {
          frame False {
            n817 = local write "ss_ceval"(FALSE ("Boolean 2")) -> ()
          }
          frame True {
            n818 = local write "ss_ceval"(TRUE ("Boolean 2")) -> ()
          }
        }
      }
      n819 = while {
        tunnel: [w522] -> w264
        tunnel: w260 -> [w521]
        tunnel: w263 -> [w520]
        tunnel: [w519] -> w262
        stop <- w518 stop-if-true
        n820 = disable-structure shown="Disabled" {
          frame Disabled {
            n821 = local read "Continue"() -> (w526:bool)
            n822 = local read "CP EV ok"() -> (w525:bool)
            n823 = local read "bypass"() -> (w524:bool)
            n824 = And(x=w526, y=w525) -> (x .and. y?=w523:bool)
            n825 = Or(x=w523, y=w524) -> ()  [unwired: 1 out]
          }
          frame Enabled {
          }
        }
        n826 = case shown="True" "teste" {
          tunnel: [w530 w533] -> w522
          tunnel: w521 -> [w531 w535]
          tunnel: w520 -> [w529 w534]
          tunnel: [w528 w532] -> w519
          frame False {
            n827 = Send Notification(notification=FALSE, notifier=w531, error in (no error)=w529) -> (notifier out=w530:refnum<notifier>, error out=w528:errorcluster)
          }
          frame True {
            n828 = local read "vec_CEVAL"() -> (w538:dbl[])
            n829 = Tick Count (ms)() -> (millisecond timer value=w537:u32)
            n830 = Tick Count (ms)() -> (millisecond timer value=w536:u32)
            n831 = while {
              shift-right: [w566] -> _
              shift-left: w538 -> [w563]
              shift-right: [w541] -> _
              shift-left: w537 -> [w540]
              shift-right: [w551] -> _
              shift-left: w536 -> [w550]
              tunnel: w535 -> [w546]
              tunnel: w534 -> [w545]
              tunnel: [w544] -> w533
              tunnel: [w543] -> w532
              stop <- w539 stop-if-true
              # "30 min"
              # "timeout ou reg permanente atingido?"
              # "Atualiza vetor de leituras"
              # "Verifica timeout"
              # "ms"
              # "ms"
              # "s"
              n832 = local read "TBR (min)"() -> (w558:u32)
              n833 = Tick Count (ms)() -> (millisecond timer value=w560:u32)
              n834 = Tick Count (ms)() -> (millisecond timer value=w557:u32)
              n835 = Multiply(x=w558, y=u32 60) -> (x*y=w567:u32)
              n836 = local read "Res_CEVAL"() -> (w564:bool)
              n837 = Subtract(x=w560, y=w550) -> (x-y=w561:u32)
              n838 = Subtract(x=w557, y=w540) -> (x-y=w559:u32)
              n839 = Multiply(x=w567, y=u32 1000) -> (x*y=w570:u32)
              n840 = Greater Or Equal?(x=w559, y=u32 1800000) -> (x >= y?=w549:bool)
              n841 = Greater Or Equal?(x=w561, y=w570) -> (x >= y?=w554:bool)
              n842 = local read "ct_CEVAL"() -> (w565:dbl)
              n843 = case shown="True" w554 {
                tunnel: w563 -> [w579 w585]
                tunnel: w565 -> [_ w587]
                tunnel: [w579 w589] -> w566
                tunnel: [w577 w588] -> w551
                tunnel: w564 -> [_ w583]
                tunnel: [FALSE w580] -> w553
                tunnel: w550 -> [w577 _]
                frame False {
                }
                frame True {
                  # "Se assentou fora da faixa do SP, reinicia vetor de leituras"
                  # "Se já possui mais de duas leituras"
                  n844 = case shown="True" w583 {
                    tunnel: [w599 w601] -> w584
                    tunnel: w585 -> [w599 _]
                    frame False {
                    }
                    frame True {
                      n845 = flat-sequence {
                        tunnel: [w602] -> w600
                        tunnel: [w604] -> w601
                        tunnel: w600 -> [w604]
                        frame #0 {
                          n846 = local read "vec_CEVAL"() -> (w602:dbl[])
                        }
                        frame #1 {
                          n847 = local write "Res_CEVAL"(FALSE ("reset")) -> ()
                        }
                      }
                    }
                  }
                  n848 = local read "PV_MIC"() -> (w582:dbl)
                  n849 = Build Array (concatenate)(w584, w582) -> (w595:dbl[])
                  n850 = call "Is Value Changed.vim"("value"=w587) -> ("changed or first call?"=w586:bool)
                  n851 = Array Subset(array=w595, index=1, length=3) -> (w589:dbl[])
                  n852 = local write "INC_CEVAL"(w586) -> ()
                  n853 = Array Max & Min(array=w589) -> (max value=w598:dbl, min value=w596:dbl)  [unwired: 2 out]
                  n854 = Greater?(x=w587, y=2) -> (0:w590:bool)
                  n855 = Subtract(x=w598, y=w596) -> (x-y=w597:dbl)
                  n856 = Less Or Equal?(x=w597, y=1.0) -> (x <= y?=w592:bool)
                  n857 = Tick Count (ms)() -> (millisecond timer value=w588:u32)
                  n858 = And(x=w590, y=w592) -> (x .and. y?=w580:bool)
                }
              }
              n859 = local read "STOP"() -> (w552:bool)
              n860 = Or(x=w552, y=w553) -> (x .or. y?=w548:bool)
              n861 = Or(x=w549, y=w548) -> (x .or. y?=w547:bool)
              n862 = call <vilib>:"Boolean Crossing PtByPt.vi"("initialize"=FALSE, "direction"=enum16{"either", "false-true", "true-false"}."false-true", "input"=w547) -> ("crossing"=w542:bool)
              n863 = Send Notification(notification=w542, notifier=w546, error in (no error)=w545) -> (notifier out=w544:refnum<notifier>, error out=w543:errorcluster)
              n864 = case shown="True" w542 {
                tunnel: [w571 w575] -> w541
                tunnel: w540 -> [w571 _]
                frame False {
                }
                frame True {
                  n865 = disable-structure shown="Disabled" {
                    frame Disabled {
                      n866 = local write "ct_CEVAL"(0.0 ("counter")) -> ()
                    }
                    frame Enabled {
                    }
                  }
                  n867 = local write "vec_CEVAL"(dbl[] [-999.0, -999.0, -999.0] ("Vetor Leituras")) -> ()
                  n868 = local write "Res_CEVAL"(TRUE ("reset")) -> ()
                  n869 = Wait (ms)(milliseconds to wait=u32 500) -> ()  [unwired: 1 out]
                  n870 = Tick Count (ms)() -> (millisecond timer value=w575:u32)
                }
              }
              n871 = local read "STOP"() -> (w539:bool)
            }
          }
        }
        n872 = local read "STOP"() -> (w518:bool)
      }
      n873 = while {
        stop <- w1514 stop-if-true
        # "PWM Generator para Chavear Relé SSR da Estufa"
        n874 = local read "Estufa_ON"() -> (w1515:bool)
        n875 = local read "STOP"() -> (w1514:bool)
        n876 = case shown="True" w1515 {
          frame False {
            n877 = Wait (ms)(milliseconds to wait=u32 100) -> ()  [unwired: 1 out]
          }
          frame True {
            w1523 = T31 0 items=["no dialog", "OK message", "continue or stop message", "OK message + warnings", "continue/stop + warnings"] ("type of dialog (OK msg:1)")
            w1534 = 10123 items=["Finite Samples"=10178, "Continuous Samples"=10123, "Hardware Timed Single Point"=12522]  # Sample Mode
            n878 = local read "Duty Cycle"() -> (w1518:sgl)
            n879 = Divide(x=w1518, y=100.0) -> (x/y=w1517:dbl)
            n880 = local read "Frequency"() -> (w1520:dbl)
            n881 = call-poly <vilib>:"DAQmx Create Virtual Channel.vi"("frequency"=w1520, "duty cycle"=w1517, "counter"=tag "Dev1/ctr3" ("Counter")) -> ("task out"=w1537:refnum<k21>, "error out"=w1536:errorcluster)  [unwired: 11 in]
            n882 = property class="DAQmx Channel"(reference=w1537, error in=w1536, "CO.Pulse.Term"=tag "/Dev1/PFI15" ("Output Terminal")) -> (reference out=w1533:refnum<k21>, error out=w1532:errorcluster)
            n883 = call-poly <vilib>:"DAQmx Timing.vi"("task/channels in"=w1533, "sample mode"=w1534, "error in"=w1532) -> ("task out"=w1531:refnum<k21>, "error out"=w1530:errorcluster)  [unwired: 11 in]
            n884 = call <vilib>:"DAQmx Start Task.vi"("task/channels in"=w1531, "error in"=w1530) -> ("task out"=w1529:refnum<k21>, "error out"=w1528:errorcluster)  [unwired: 12 in]
            n885 = while {
              tunnel: w1529 -> [w1548]
              tunnel: w1528 -> [w1546]
              tunnel: [w1557] -> w1525
              tunnel: [w1558] -> w1526
              tunnel: [FALSE ("Liga aquecedor")] -> w1522
              tunnel: w1517 -> [w1544]
              tunnel: w1520 -> [w1542]
              stop <- w1551 stop-if-true
              # "era F"
              n886 = local read "Duty Cycle"() -> (w1541:sgl)
              n887 = Wait Until Next ms Multiple(millisecond multiple=u32 10) -> ()  [unwired: 1 out]
              n888 = Divide(x=w1541, y=100.0) -> (x/y=w1539:dbl)
              n889 = Not Equal?(x=w1544, y=w1539) -> (x != y?=w1543:bool)
              n890 = case shown="True" w1543 {
                tunnel: [w1560 w1563] -> w1547
                tunnel: w1548 -> [w1560 w1564]
                tunnel: [w1559 w1565] -> w1545
                tunnel: w1546 -> [w1559 w1566]
                tunnel: w1539 -> [_ w1562]
                tunnel: w1542 -> [_ w1561]
                frame False {
                }
                frame True {
                  n891 = call-poly <vilib>:"DAQmx Write.vi"("task/channels in"=w1564, "frequency"=w1561, "duty cycle"=w1562, "error in"=w1566) -> ("task out"=w1563:refnum<k21>, "error out"=w1565:errorcluster)  [unwired: 9 in, 1 out]
                }
              }
              n892 = call <vilib>:"DAQmx Is Task Done.vi"("task/channels in"=w1547, "error in"=w1545) -> ("task out"=w1558:refnum<k21>, "error out"=w1557:errorcluster)  [unwired: 11 in, 1 out]
              n893 = local read "Estufa_ON"() -> (w1554:bool)
              n894 = Unbundle By Name(w1557) -> ("status"=w1556:bool)
              n895 = Not(x=w1554) -> (.not. x?=w1552:bool)
              n896 = local read "STOP"() -> (w1549:bool)
              n897 = Or(x=w1556, y=w1552) -> (x .or. y?=w1550:bool)
              n898 = Or(x=w1550, y=w1549) -> (x .or. y?=w1551:bool)
            }
            n899 = call <vilib>:"DAQmx Stop Task.vi"("task/channels in"=w1526, "error in"=w1525) -> ("task out"=w1521:refnum<k21>, "error out"=w1527:errorcluster)  [unwired: 12 in]
            n900 = local write "Estufa_ON"(w1522) -> ()
            n901 = call <vilib>:"DAQmx Clear Task.vi"("task in"=w1521, "error in"=w1527) -> ("error out"=w1524:errorcluster)  [unwired: 13 in]
            n902 = call <vilib>:"Simple Error Handler.vi"("error code (no error:0)"=w1523, "error in (no error)"=w1524) -> ()  [unwired: 3 in, 5 out]
          }
        }
      }
      n903 = while {
        stop <- w371 stop-if-true
        n904 = local read "LIM SS MF"() -> (w374:bool)
        n905 = local read "STEADY MF?"() -> (w373:bool)
        n906 = local read "STOP"() -> (w371:bool)
        n907 = Not(x=w374) -> (.not. x?=w372:bool)
        n908 = And(x=w373, y=w372) -> (x .and. y?=w375:bool)
        n909 = case shown="True" w375 {
          frame False {
          }
          frame True {
            n910 = local write "vecTempME"(dbl[] [-999.0, -999.0, -999.0] ("Vetor Leituras")) -> ()
            n911 = local write "Res_TempME"(TRUE ("reset")) -> ()
          }
        }
      }
      n912 = Obtain Queue(name (unnamed)="comando", element data type=TRUE, create if not found? (T)=TRUE) -> (queue out=w255:refnum<queue>)  [unwired: 2 in, 2 out]
      n913 = while {
        tunnel: w255 -> [w492]
        tunnel: [w492] -> w254
        stop <- w493 stop-if-true
        n914 = property on="Condicao para teste" class="Enum (strict)"() -> ("Strings []"=w495:string[])  [unwired: 2 in, 2 out]
        n915 = local read "STOP"() -> (w493:bool)
        n916 = Array Size(array=w495) -> (size(s)=w494:i32)
        n917 = while {
          tunnel: w494 -> [w499]
          tunnel: w492 -> [w496]
          stop <- w497 stop-if-true
          # "quantas condicoes de teste?"
          # "Controle da Condicao de Operacao do Teste Comp Eval"
          n918 = for {
            N: w499 -> [_]
            tunnel: w496 -> [w500]
            i -> [w501]
            n919 = property on="Condicao para teste" class="Enum (strict)"("Value"=w501) -> ()  [unwired: 2 in, 2 out]
            n920 = while {
              tunnel: w500 -> [w509]
              stop <- w506 stop-if-true
              # "Se a temperatura do componente assentou,o sistema pode partir para a proxima condicao de ensaio (potencia e velocidade)"
              n921 = property on="Condicao para teste" class="Enum (strict)"() -> ("RingText.Text"=w510:string)  [unwired: 2 in, 2 out]
              "Condição Atual" <- w510
              n922 = local read "ss_ceval"() -> (w504:bool)
              n923 = local read "STOP"() -> (w502:bool)
              n924 = Scan From String(format string="%dRPM@%dW", input string=w510) -> (output 1=→"SP_Vel":i32, output 2=→"SP_Pwr":i32)  [unwired: 4 in, 3 out]
              n925 = Or(x="Skip", y=w504) -> (x .or. y?=w503:bool)
              n926 = case shown="True" w503 {
                selector: w503 -> [_ w514]
                tunnel: w509 -> [_ w516]
                tunnel: [FALSE w514] -> w508
                frame False {
                }
                frame True {
                  # "era 1000"
                  n927 = Enqueue Element(queue=w516, element=w514) -> ()  [unwired: 2 in, 3 out]
                  n928 = Wait (ms)(milliseconds to wait=u32 1000) -> ()  [unwired: 1 out]
                }
              }
              n929 = Or(x=w508, y=w502) -> (x .or. y?=w506:bool)
            }
            "iter" <- w501
          }
          n930 = local read "iter"() -> (w498:i32)
          n931 = Less Or Equal?(x=w498, y=w499) -> (x <= y?=w497:bool)
        }
      }
      n932 = while {
        stop <- w1012 stop-if-true
        # "Modo Manual"
        # "Modo Power Map"
        # "Malha Externa Externa - Controle de Temperatura por Restrição - Override Control Min Selector"
        n933 = local read "PW MP ok"() -> (w1010:bool)
        n934 = local read "Manual"() -> (w1011:bool)
        n935 = Not(x=w1011) -> (.not. x?=w1009:bool)
        n936 = And(x=w1010, y=w1009) -> (x .and. y?=w1008:bool)
        n937 = case shown="True" w1008 {
          frame False {
            # "Modo manual ligado, referencia de potencia da malha externa é zero"
            n938 = local read "Ts ME"() -> (w1015:dbl)
            n939 = Multiply(x=w1015, y=u32 1000 ("milliseconds to wait")) -> (x*y=w1014:dbl)
            n940 = local read "TP 13"() -> (w1019:dbl)
            n941 = local read "TP 12"() -> (w1018:dbl)
            n942 = local read "TP 1"() -> (w1016:dbl)
            n943 = local read "TP 10"() -> (w1017:dbl)
            n944 = local write "MV_ME"(sgl 0.0 ("MV_ME")) -> ()
            n945 = Wait (ms)(milliseconds to wait=w1014) -> ()  [unwired: 1 out]
            n946 = Bundle("TP 1"=w1016, "TP 10"=w1017, "TP 12"=w1018, "TP 13"=w1019) -> (w1020:T32)  [unwired: 1 in]
            n947 = local write "SPs_Filtro"(w1020) -> ()
          }
          frame True {
            w1053 = cluster{"output high":dbl, "output low":dbl} {"output high"=900.0, "output low"=0.0} ("output range")
            # "zero do filtro"
            # "Modo manual desacionado e power map habilitado, executa malha externa com controle override min"
            n948 = local read "zF_C5"() -> (w1023:dbl)
            n949 = local read "zF_L1"() -> (w1024:dbl)
            n950 = local read "zF_C1"() -> (w1025:dbl)
            n951 = local read "TP 13"() -> (w1028:dbl)
            n952 = local read "TP 10"() -> (w1035:dbl)
            n953 = local read "TP 12"() -> (w1031:dbl)
            n954 = local read "TP 1"() -> (w1040:dbl)
            n955 = local read "zF_MIC"() -> (w1022:dbl)
            n956 = local write "zF_C1_i"(w1025) -> ()
            n957 = local write "zF_C5_i"(w1023) -> ()
            n958 = local write "zF_L1_i"(w1024) -> ()
            n959 = Multiply(x="Ts ME", y=u32 1000 ("milliseconds to wait")) -> (x*y=w1058:dbl)
            n960 = Wait Until Next ms Multiple(millisecond multiple=w1058) -> ()  [unwired: 1 out]
            n961 = local write "zF_MIC_i"(w1022) -> ()
            n962 = feedback #1(0.0) -> (w1049:dbl)
            n963 = call "pid_erf.vi"("process variable"=w1040, "output range"=w1053, "PID gains"="Gains_C1", "alfa"=w1025, "dt (s)"="Ts ME", "setpoint"="SP_C1", "erf"=w1049) -> ("output"=w1044:dbl, "SP_F"=w1039:dbl)  [unwired: 2 in, 1 out]
            n964 = call "pid_erf.vi"("process variable"=w1035, "output range"=w1053, "PID gains"="Gains_L1", "alfa"=w1024, "dt (s)"="Ts ME", "setpoint"="SP_L1", "erf"=w1049) -> ("output"=w1043:dbl, "SP_F"=w1034:dbl)  [unwired: 2 in, 1 out]
            n965 = call "pid_erf.vi"("process variable"=w1031, "output range"=w1053, "PID gains"="Gains_C5", "alfa"=w1023, "dt (s)"="Ts ME", "setpoint"="SP_C5", "erf"=w1049) -> ("output"=w1042:dbl, "SP_F"=w1027:dbl)  [unwired: 2 in, 1 out]
            n966 = call "pid_erf.vi"("process variable"=w1028, "output range"=w1053, "PID gains"="Gains_MIC", "alfa"=w1022, "dt (s)"="Ts ME", "setpoint"="SP_MIC", "erf"=w1049) -> ("output"=w1045:dbl, "SP_F"=w1026:dbl)  [unwired: 2 in, 1 out]
            n967 = Bundle("SP_F"=w1039, "SP_F"=w1034, "SP_F"=w1027, "SP_F"=w1026) -> (w1046:T1)  [unwired: 1 in]
            n968 = Bundle("SP_C1"="SP_C1", "TP 1"=w1040, "SP_F"=w1039) -> (w1038:cluster{"SP_C1":dbl, "TP 1":dbl, "SP_F":dbl})  [unwired: 1 in]
            n969 = Bundle("SP_L1"="SP_L1", "TP 10"=w1035, "SP_F"=w1034) -> (w1037:cluster{"SP_L1":dbl, "TP 10":dbl, "SP_F":dbl})  [unwired: 1 in]
            n970 = Bundle("SP_C5"="SP_C5", "TP 12"=w1031, "SP_F"=w1027) -> (w1033:cluster{"SP_C5":dbl, "TP 12":dbl, "SP_F":dbl})  [unwired: 1 in]
            n971 = Bundle("SP_MIC"="SP_MIC", "TP 13"=w1028, "SP_F"=w1026) -> (w1030:cluster{"SP_MIC":dbl, "TP 13":dbl, "SP_F":dbl})  [unwired: 1 in]
            n972 = local write "SPs_Filtro"(w1046) -> ()
            n973 = local write "GME_C1"(w1038) -> ()
            n974 = local write "GME_L1"(w1037) -> ()
            n975 = local write "GME_C5"(w1033) -> ()
            n976 = local write "GME_MIC"(w1030) -> ()
            n977 = local write "MV_MIC"(w1045) -> ()
            n978 = Build Array(w1044, w1043, w1042, w1045) -> (w1051:dbl[])
            n979 = local write "MV_C1"(w1044) -> ()
            n980 = local write "MV_C5"(w1042) -> ()
            n981 = local write "MV_L1"(w1043) -> ()
            n982 = Array Max & Min(array=w1051) -> (min value=w1047:dbl)  [unwired: 3 out]
            n983 = feedback-in #1(w1047) -> ()
            n984 = local write "Graf_MV_MIC"(w1045) -> ()
            n985 = local write "Graf_MV_C1"(w1044) -> ()
            n986 = local write "Graf_MV_C5"(w1042) -> ()
            n987 = local write "Graf_MV_L1"(w1043) -> ()
            n988 = local write "MV_ME"(w1047) -> ()
          }
        }
        n989 = local read "STOP"() -> (w1012:bool)
      }
      n990 = while {
        stop <- w889 stop-if-true
        # "velocidade atualizou?"
        # "Se está em modo manual, a corrente do freio é setada pelo operador na IHM"
        # "Satura corrente de saída"
        # "Modo auto?"
        # "Potencia de saída da malha interna"
        # "Modo Component Eval"
        # "corrente aplicada ao freio"
        # "ms"
        # "Gain scheduling PID - Malha Interna - Controle de Potência"
        n991 = local read "SP_Vel"() -> (w878:i32)
        n992 = local read "CP EV ok"() -> (w880:bool)
        n993 = call "Is Value Changed.vim"("value"=w878) -> ("changed or first call?"=w877:bool)
        n994 = case shown="True" "bypass" {
          selector: "bypass" -> [_ w899]
          tunnel: [w898 w900] -> w879
          frame False {
            n995 = local read "Manual"() -> (w898:bool)
          }
          frame True {
            w901 = FALSE ("Manual")
            n996 = local write "Manual"(w901) -> ()
            n997 = local write "Seta carga"(w901) -> ()
            n998 = Not(x=w899) -> (.not. x?=w900:bool)
          }
        }
        n999 = Or(x="bypass", y=w880) -> (x .or. y?=w876:bool)
        n1000 = And(x=w876, y=w877) -> (x .and. y?=w875:bool)
        n1001 = case shown="False" w876 {
          tunnel: [w902 w903] -> w871
          frame True {
            # "SP de potencia vem da Comp Eval"
            n1002 = local read "SP_Pwr"() -> (w902:i32)
          }
          frame False {
            # "SP Potencia vem da malha externa"
            # "Cascata On"
            n1003 = local read "MV_ME"() -> (w903:sgl)
          }
        }
        n1004 = case shown="True" w875 {
          frame False {
          }
          frame True {
            n1005 = local read "Parâmetros serial"() -> (w896:T10)
            n1006 = local read "SP_Vel"() -> (w894:i32)
            n1007 = call "Serial_control.vi"("Enviar número"=w894, "Função"=T21."Set Speed", "comm cluster"=w896) -> ("translated message"=w895:string)  [unwired: 2 in, 3 out]
            n1008 = local write "Tradução"(w895) -> ()
          }
        }
        n1009 = local read "PV_MI"() -> (w872:dbl)
        n1010 = call-poly <vilib>:"PID Gain Schedule.vi"("PID gain schedule"="Ganhos PI do Gain Scheduling", "gain scheduling value"=w872) -> ("PID gains out"=w892:T3)  [unwired: 2 in, 1 out]
        "Ganho atual do PI MI" <- w892
        n1011 = Bundle("PV_MI"=w872, "MV_ME"=w871) -> (→"Grafico_MI":cluster{"PV_MI":dbl, "MV_ME":sgl})  [unwired: 1 in]
        n1012 = Not(x=w879) -> (.not. x?=w886:bool)
        n1013 = local read "Limite de corrente"() -> (w887:dbl)
        n1014 = Multiply(x="Ts MI", y=1000.0) -> (x*y=w891:dbl)
        n1015 = Wait Until Next ms Multiple(millisecond multiple=w891) -> ()  [unwired: 1 out]
        n1016 = call-poly <vilib>:"PID Advanced.vi"("setpoint"=w871, "output range"=cluster{"output high":dbl, "output low":dbl} {"output high"=0.31, "output low"=0.0}, "auto? (T)"=w886, "manual control"=w887, "process variable"=w872, "PID gains"=w892, "dt (s)"="Ts MI") -> ("output"=w873:dbl)  [unwired: 7 in, 1 out]
        "MV_MI" <- w873
        "Graf_MV_MI" <- w873
        n1017 = call <instrlib>:"GENie Config Current Limit.vi"("Current Limit"=w873, "VISA"=refnum<visa-resource-name> "Lambda" ("VISA name")) -> ("error out"=w883:errorcluster)  [unwired: 8 in, 1 out]
        n1018 = Unbundle By Name(w883) -> ("code"=w884:i32)
        n1019 = local read "STOP"() -> (w889:bool)
        n1020 = call <vilib>:"Clear Errors.vi"("specific error code to clear (0: all)"=w884) -> ()  [unwired: 5 in, 2 out]
      }
      n1021 = while {
        shift-right: [w364] -> _
        shift-left: 0.0 -> [w363]
        stop <- w361 stop-if-true
        # "Contador de leituras do vector de temps da estufa"
        n1022 = local read "INC_TempME"() -> (w362:bool)
        n1023 = local read "STOP"() -> (w361:bool)
        n1024 = case shown="True" w362 {
          tunnel: [w365 w367] -> w364
          tunnel: w363 -> [w365 w366]
          frame False {
          }
          frame True {
            n1025 = flat-sequence {
              tunnel: w366 -> [w369]
              tunnel: [w368] -> w367
              frame #0 {
                n1026 = Increment(x=w369) -> (x+1=w368:dbl)
                n1027 = local write "ct_TempME"(w368) -> ()
              }
              frame #1 {
                n1028 = local write "INC_TempME"(FALSE ("increment")) -> ()
              }
            }
          }
        }
      }
      n1029 = disable-structure shown="Disabled" {
        disable-tunnel: w268 -> [w607 _]
        disable-tunnel: w267 -> [w606 _]
        disable-tunnel: [w605 _] -> w269
        frame Disabled {
          n1030 = call <instrlib>:"Close.vi"("error in (no error)"=w606, "VISA resource name"=w607) -> ("error out"=w605:errorcluster)  [unwired: 9 in]
        }
        frame Enabled {
        }
      }
      n1031 = call <instrlib>:"Close.vi"("error in (no error)"=w272, "VISA resource name"=w273) -> ()  [unwired: 9 in, 1 out]
      n1032 = Release Notifier(notifier=w264, error in (no error)=w262) -> ()  [unwired: 1 in, 3 out]
      n1033 = Release Notifier(notifier=w248, error in (no error)=w247) -> ()  [unwired: 1 in, 3 out]
      n1034 = call <vilib>:"Simple Error Handler.vi"("error in (no error)"=w269) -> ()  [unwired: 4 in, 5 out]
      n1035 = Release Queue(queue=w254) -> ()  [unwired: 2 in, 3 out]
    }
    frame #2 {
      n1036 = local write "STOP"(FALSE ("STOP")) -> ()
    }
  }
  n1037 = disable-structure shown="Disabled" {
    frame Disabled {
      # "Inicia vetor"
      # "Inicia vetor"
      n1038 = Tick Count (ms)() -> (millisecond timer value=w1593:u32)
      n1039 = Tick Count (ms)() -> (millisecond timer value=w1590:u32)
      n1040 = Initialize Array(-999.0 ("element"), 3 ("dimension size")) -> (w1592:dbl[])
      n1041 = Initialize Array(-999.0 ("element"), 3 ("dimension size")) -> (w1591:dbl[])
      n1042 = while {
        shift-right: [w1598] -> _
        shift-left: w1592 -> [w1609]
        shift-right: [w1602] -> _
        shift-left: w1593 -> [w1601]
        i -> [w1608]
        stop <- w1596 stop-if-true
        # "Atualiza"
        # "ms"
        # "ms"
        # "s"
        # "Verifica se a temperatura do componente controlado atingiu o regime permanente"
        n1043 = local read "TBRMF(min)"() -> (w1594:u32)
        n1044 = Tick Count (ms)() -> (millisecond timer value=w1604:u32)
        n1045 = Multiply(x=w1594, y=u32 60) -> (x*y=w1599:u32)
        n1046 = Subtract(x=w1604, y=w1601) -> (x-y=w1605:u32)
        n1047 = Multiply(x=w1599, y=u32 1000) -> (x*y=w1607:u32)
        n1048 = Greater Or Equal?(x=w1605, y=w1607) -> (x >= y?=w1603:bool)
        n1049 = case shown="True" w1603 {
          tunnel: [FALSE w1631] -> w1597
          tunnel: w1609 -> [w1611 w1630]
          tunnel: w1608 -> [w1612 w1625]
          tunnel: [w1611 w1622] -> w1598
          tunnel: [w1610 w1621] -> w1602
          tunnel: w1601 -> [w1610 _]
          frame False {
            n1050 = disable-structure shown="Disabled" {
              disable-tunnel: w1612 -> [w1614 _]
              frame Disabled {
              }
              frame Enabled {
              }
            }
          }
          frame True {
            w1619 = 1.0 ("y")
            # "Se já possui mais de duas leituras"
            # "Esta dentro da faixa desejada?"
            # "Se sim para os dois casos,\nentao a temperatura atingiu\nseu limite"
            # "Entrou em regime permanente?"
            n1051 = local read "PV_MIC"() -> (w1620:dbl)
            n1052 = Build Array (concatenate)(w1630, w1620) -> (w1629:dbl[])
            n1053 = Array Subset(array=w1629, index=1, length=3) -> (w1622:dbl[])
            n1054 = Array Max & Min(array=w1622) -> (max value=w1640:dbl, min value=w1638:dbl)  [unwired: 2 out]
            n1055 = local read "SP_MIC"() -> (w1618:dbl)
            n1056 = Greater?(x=w1625, y=2) -> (0:w1623:bool)
            n1057 = Subtract(x=w1640, y=w1638) -> (x-y=w1639:dbl)
            n1058 = local read "PV_MIC"() -> (w1636:dbl)
            n1059 = Add(x=w1618, y=w1619) -> (x+y=w1634:dbl)
            n1060 = Subtract(x=w1618, y=w1619) -> (x-y=w1635:dbl)
            n1061 = Greater Or Equal?(x=w1636, y=w1635) -> (x >= y?=w1633:bool)
            n1062 = Less Or Equal?(x=w1636, y=w1634) -> (x <= y?=w1632:bool)
            n1063 = Less Or Equal?(x=w1639, y=w1619) -> (x <= y?=w1626:bool)
            n1064 = And(x=w1632, y=w1633) -> (x .and. y?=w1637:bool)
            n1065 = And(x=w1623, y=w1626) -> (x .and. y?=w1616:bool)
            n1066 = local read "STOP"() -> (w1617:bool)
            n1067 = And(x=w1616, y=w1637) -> (x .and. y?=w1615:bool)
            n1068 = local write "STEADY MF?"(w1616) -> ()
            n1069 = local write "LIM SS MF"(w1615) -> ()
            n1070 = Or(x=w1615, y=w1617) -> (x .or. y?=w1631:bool)
            n1071 = Tick Count (ms)() -> (millisecond timer value=w1621:u32)
          }
        }
        n1072 = local read "STOP"() -> (w1595:bool)
        n1073 = Or(x=w1597, y=w1595) -> (x .or. y?=w1596:bool)
      }
      n1074 = while {
        shift-right: [w1645] -> _
        shift-left: w1591 -> [w1656]
        shift-right: [w1649] -> _
        shift-left: w1590 -> [w1648]
        i -> [w1655]
        stop <- w1643 stop-if-true
        # "Atualiza"
        # "ms"
        # "ms"
        # "s"
        # "Verifica se a temperatura do componente controlado atingiu o regime permanente"
        n1075 = local read "TBRMF(min)"() -> (w1641:u32)
        n1076 = Tick Count (ms)() -> (millisecond timer value=w1651:u32)
        n1077 = Multiply(x=w1641, y=u32 60) -> (x*y=w1646:u32)
        n1078 = Subtract(x=w1651, y=w1648) -> (x-y=w1652:u32)
        n1079 = Multiply(x=w1646, y=u32 1000) -> (x*y=w1654:u32)
        n1080 = Greater Or Equal?(x=w1652, y=w1654) -> (x >= y?=w1650:bool)
        n1081 = case shown="True" w1650 {
          tunnel: [FALSE w1678] -> w1644
          tunnel: w1656 -> [w1658 w1677]
          tunnel: w1655 -> [w1659 w1672]
          tunnel: [w1658 w1669] -> w1645
          tunnel: [w1657 w1668] -> w1649
          tunnel: w1648 -> [w1657 _]
          frame False {
            n1082 = disable-structure shown="Disabled" {
              disable-tunnel: w1659 -> [w1661 _]
              frame Disabled {
              }
              frame Enabled {
              }
            }
          }
          frame True {
            w1666 = 1.0 ("y")
            # "Se já possui mais de duas leituras"
            # "Esta dentro da faixa desejada?"
            # "Se sim para os dois casos,\nentao a temperatura atingiu\nseu limite"
            # "Entrou em regime permanente?"
            n1083 = local read "PV_MIC"() -> (w1667:dbl)
            n1084 = Build Array (concatenate)(w1677, w1667) -> (w1676:dbl[])
            n1085 = Array Subset(array=w1676, index=1, length=3) -> (w1669:dbl[])
            n1086 = Array Max & Min(array=w1669) -> (max value=w1687:dbl, min value=w1685:dbl)  [unwired: 2 out]
            n1087 = local read "SP_MIC"() -> (w1665:dbl)
            n1088 = Greater?(x=w1672, y=2) -> (0:w1670:bool)
            n1089 = Subtract(x=w1687, y=w1685) -> (x-y=w1686:dbl)
            n1090 = local read "PV_MIC"() -> (w1683:dbl)
            n1091 = Add(x=w1665, y=w1666) -> (x+y=w1681:dbl)
            n1092 = Subtract(x=w1665, y=w1666) -> (x-y=w1682:dbl)
            n1093 = Greater Or Equal?(x=w1683, y=w1682) -> (x >= y?=w1680:bool)
            n1094 = Less Or Equal?(x=w1683, y=w1681) -> (x <= y?=w1679:bool)
            n1095 = Less Or Equal?(x=w1686, y=w1666) -> (x <= y?=w1673:bool)
            n1096 = And(x=w1679, y=w1680) -> (x .and. y?=w1684:bool)
            n1097 = And(x=w1670, y=w1673) -> (x .and. y?=w1663:bool)
            n1098 = local read "STOP"() -> (w1664:bool)
            n1099 = And(x=w1663, y=w1684) -> (x .and. y?=w1662:bool)
            n1100 = local write "STEADY MF?"(w1663) -> ()
            n1101 = local write "LIM SS MF"(w1662) -> ()
            n1102 = Or(x=w1662, y=w1664) -> (x .or. y?=w1678:bool)
            n1103 = Tick Count (ms)() -> (millisecond timer value=w1668:u32)
          }
        }
        n1104 = local read "STOP"() -> (w1642:bool)
        n1105 = Or(x=w1644, y=w1642) -> (x .or. y?=w1643:bool)
      }
    }
    frame Enabled {
    }
  }
